vi "STD Cal Data_etc.vi"(8 "error in":errorcluster caption="에러 입력(에러 없음)", 9 "Data in":string[][](array[string]), 10 "문자열":string, 11 "Func_ext":string) -> (0 "error out":errorcluster caption="에러 출력", 1 "Data Out":string[][](array[string]), 3 "Func_ext Out":string, 4 "Data Out 2":string[](array[string]), 6 "Cal STD":string[][](array[string]))   [LabVIEW 2020]
uses:
  Controls/Cmd_Var Data IO.ctl
  Controls/Cmd_File path.ctl
  Controls/Cmd_File Type.ctl
  Variables/Global_Cal STD.vi
  Variables/Global_Cal Info.vi
  Public/Polymorph/Array Dedup_2D Str.vi
  Public/Polymorph/Data Class_2D Str.vi
  Public/Polymorph/Sort_2D Str.vi
  <vilib>/Utility/file.llb/Read Delimited Spreadsheet (string).vi
  Public/Polymorph/Array Dedup_1D Str.vi
panel:
  out "Cal STD in":string[][](array[string])
  out "Condition Default":string[][](array[string])
  out "데이터오류?":bool
  out "생성오류?":bool
  out "Condition":string[][](array[string])
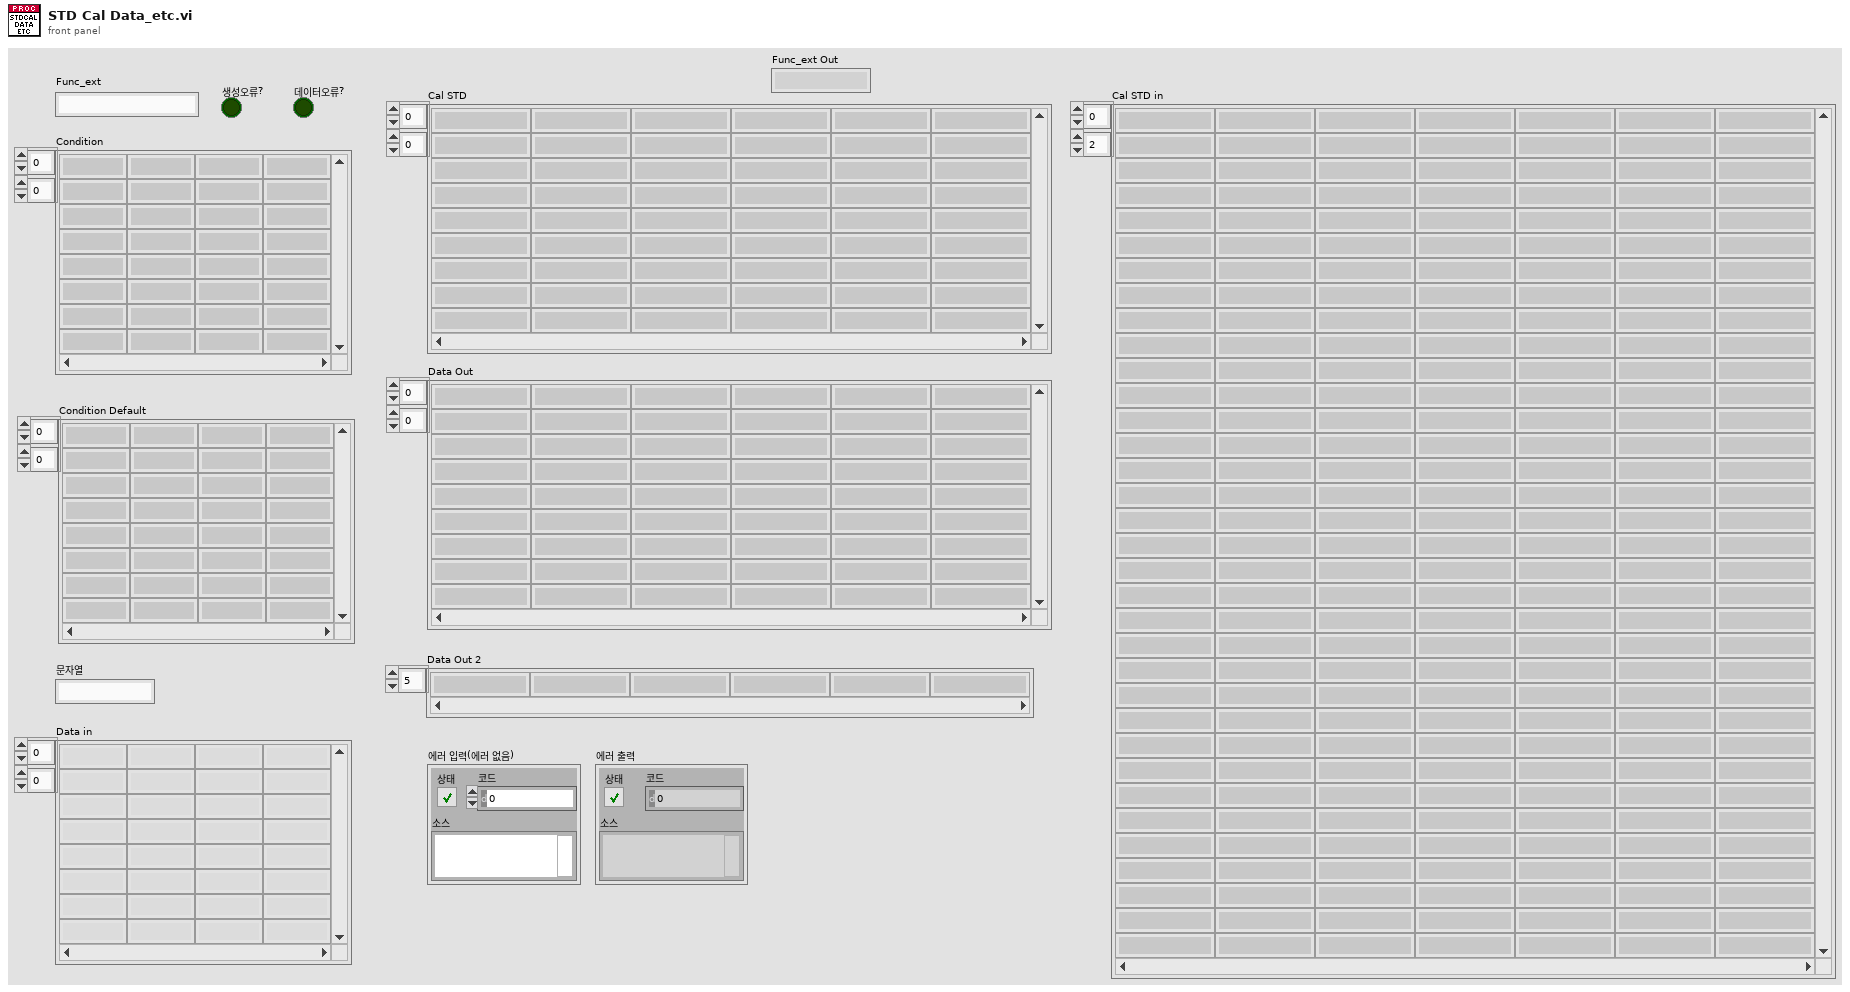
[diagram p1: front panel]
types:
  T1 = typedef "Cmd_Var Data IO.ctl" = enum16{"Condition", "Condition Default", "Condition_Temp", "Resolution", "Resolution Default", "Resolution Old", "Spec", "Spec Default", "Spec Old", "Spec Temp", "Result", "Result2", "Result3", "Result_Temp", "Result_ADJ", "Result_ADJ2", "STD1", "STD2", "STD3", "STD4", "STD5", "STD Temp", "CMC", "CMC Default"}
  T2 = cluster{"세부분류코드":string, "형식":string, "옵션":string, "측정기명":string, "EXCEL파일명":string, "TEMP":string}
  T3 = typedef "Cmd_File Type.ctl" = enum16{"엑셀", "엑셀(2003)", "텍스트", "설정", "2진", "VI", "CSV", "LOG", "폴더"}
  T4 = typedef "Cmd_File path.ctl" = enum16{"에러로그", "데이터파일경로", "성적서원본", "지난성적서", "Data Files", "경로생성", "Updater", "Template", "설정파일경로", "FTP Upload", "Update 경로", "어플리케이션"}
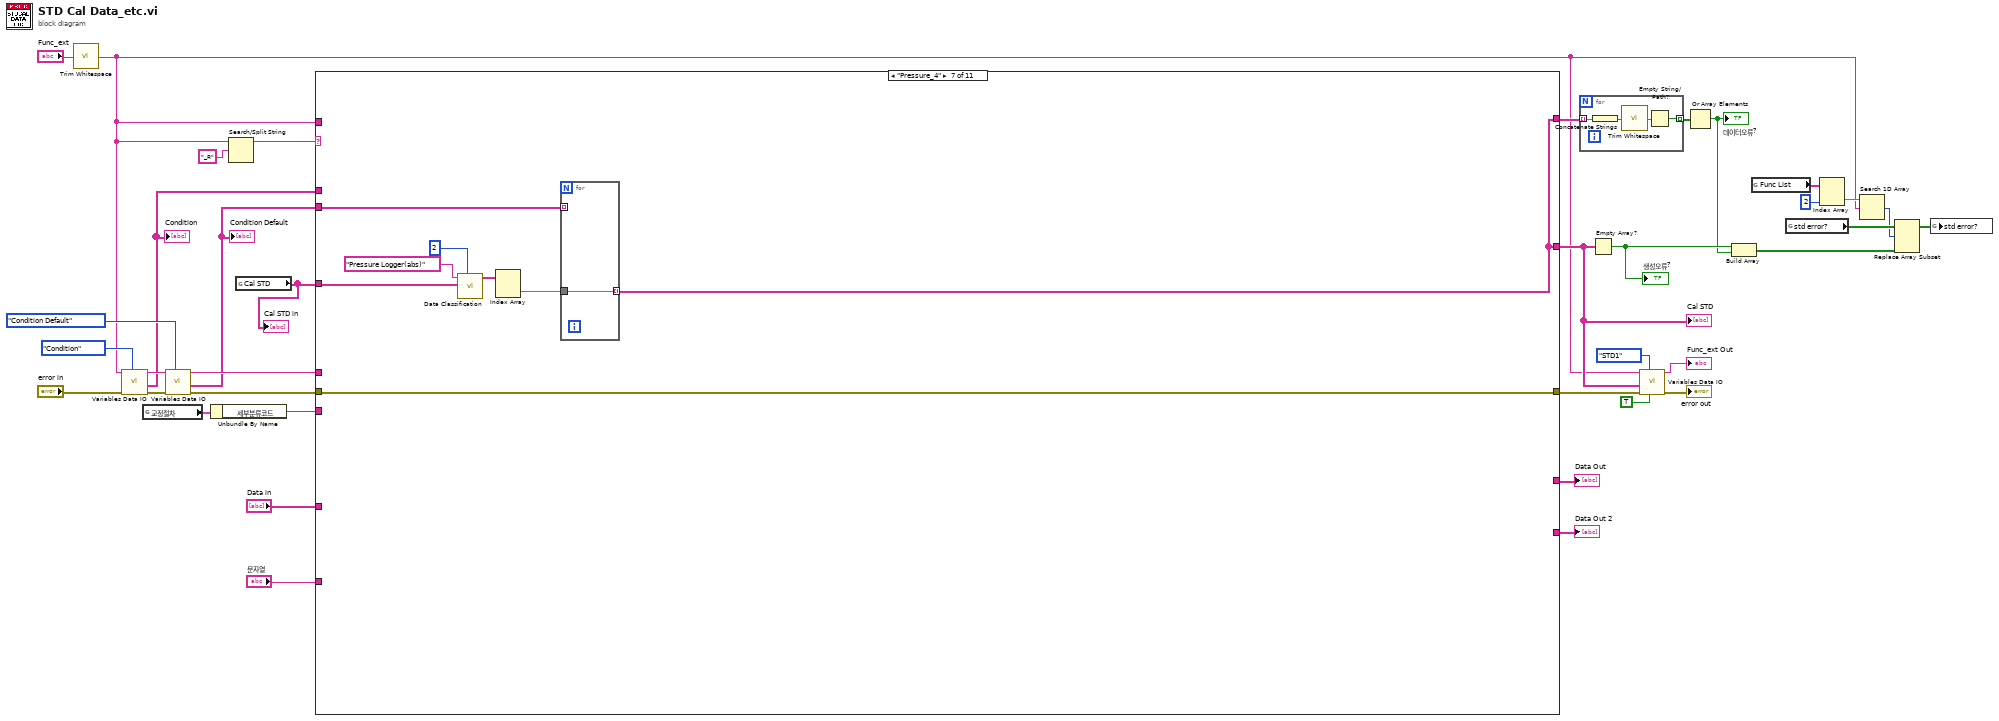
[diagram p0: block diagram]
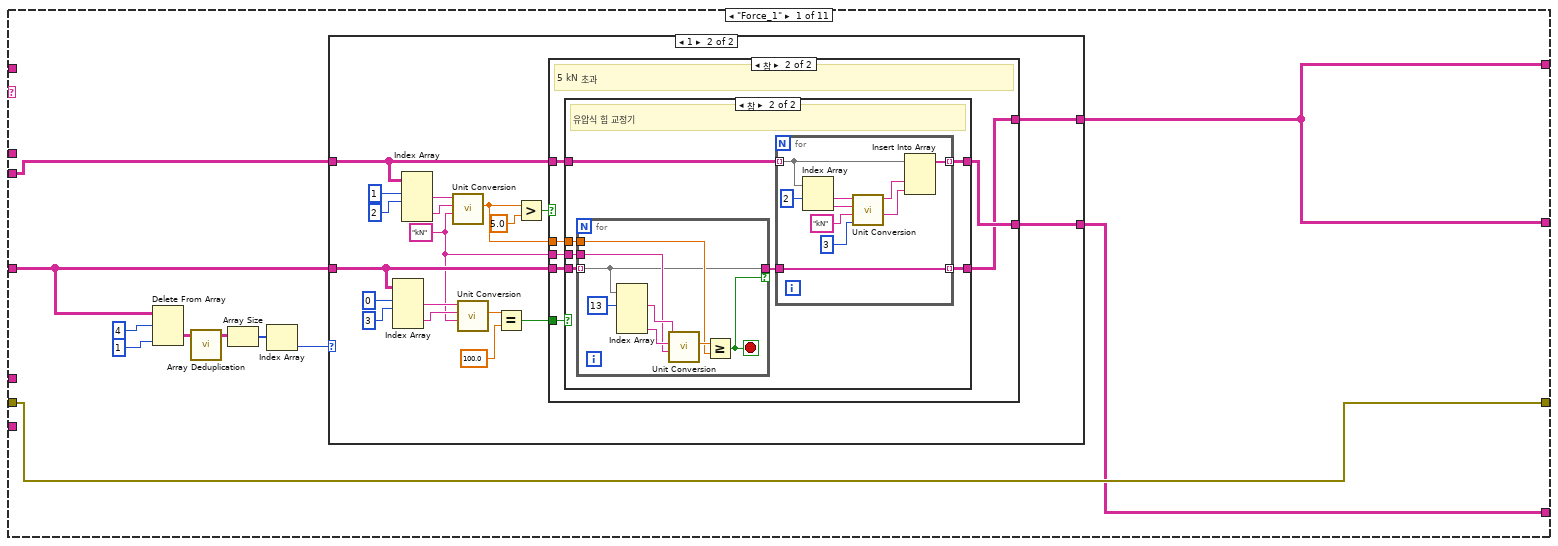
[diagram p2: hidden frame]
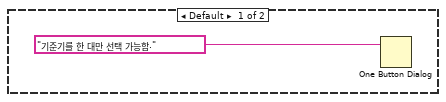
[diagram p3: hidden frame]
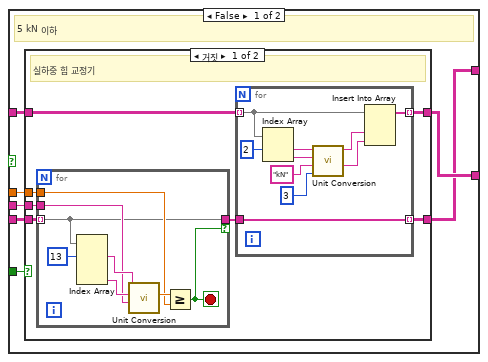
[diagram p4: hidden frame]
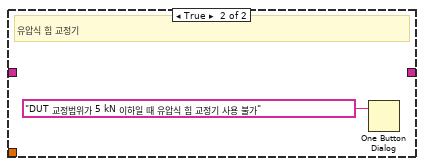
[diagram p5: hidden frame]
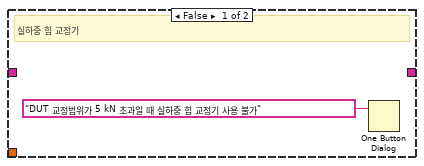
[diagram p6: hidden frame]
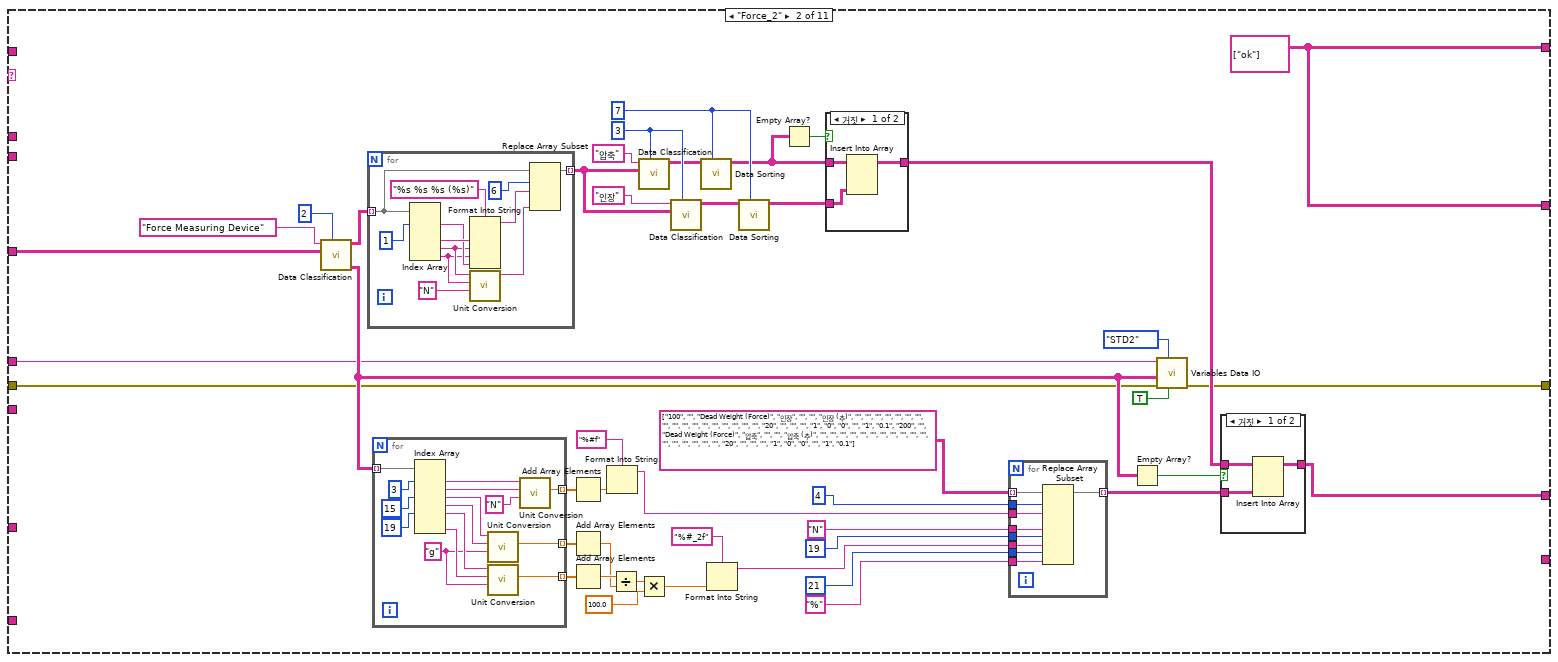
[diagram p7: hidden frame]
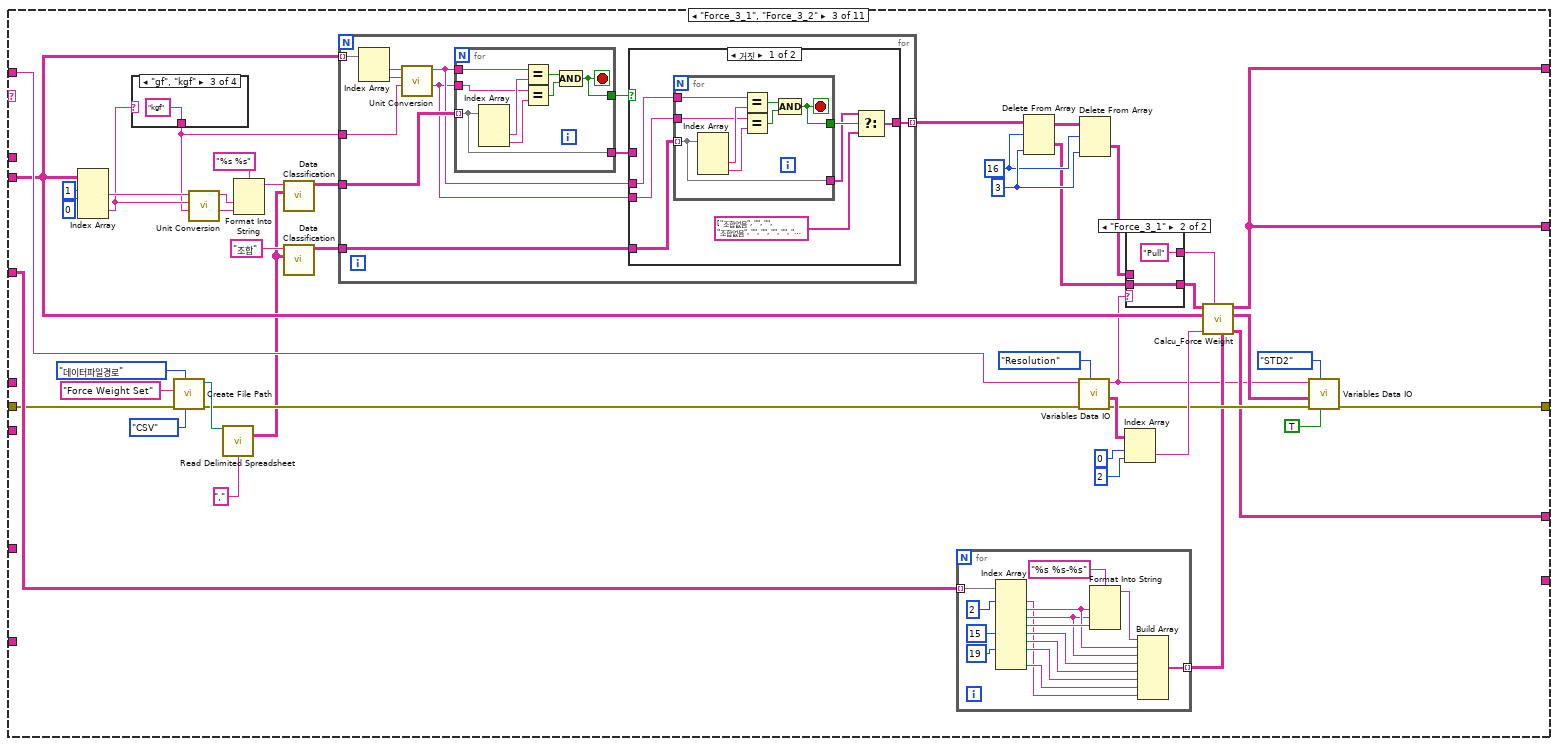
[diagram p10: hidden frame]
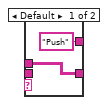
[diagram p11: hidden frame]
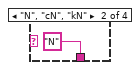
[diagram p14: hidden frame]
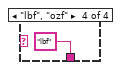
[diagram p15: hidden frame]
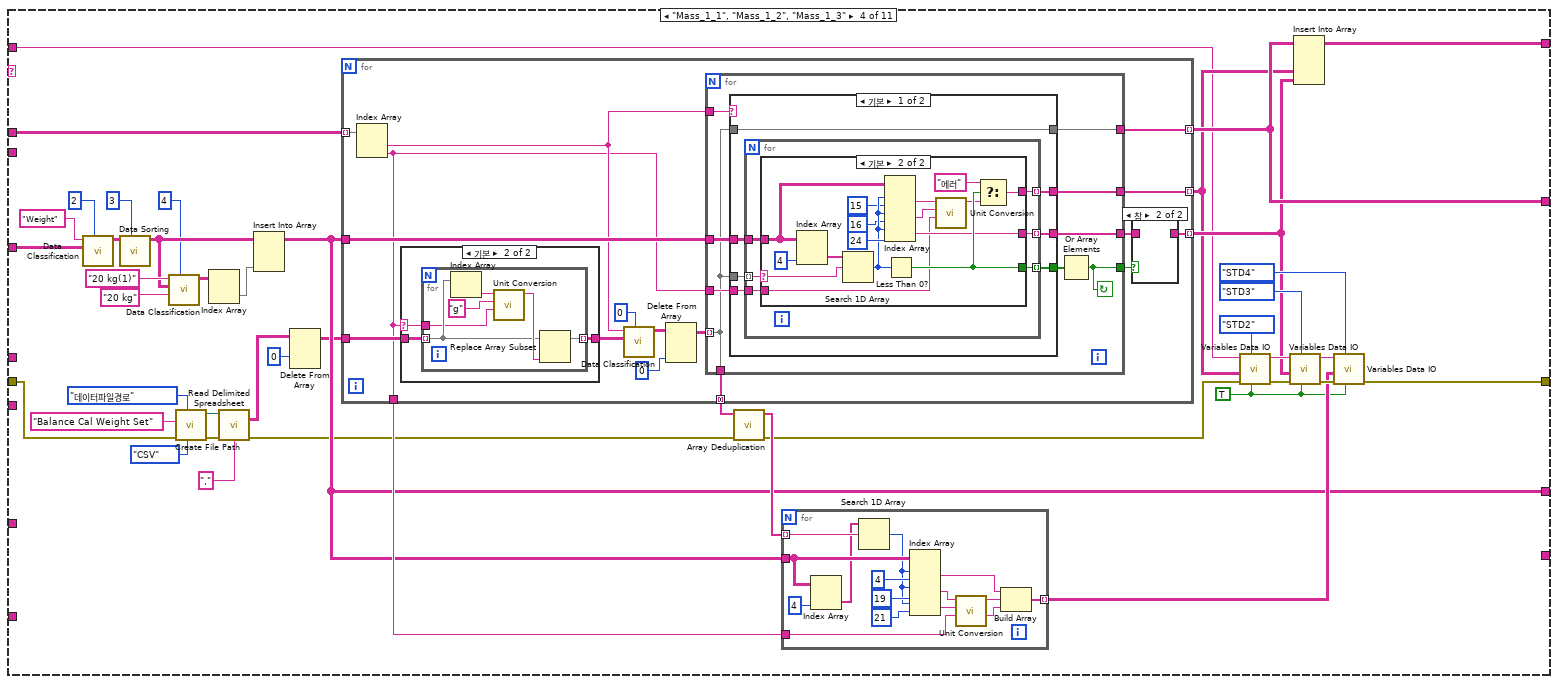
[diagram p16: hidden frame]
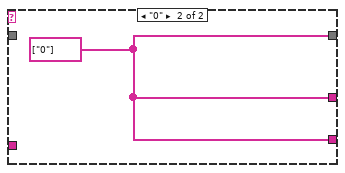
[diagram p19: hidden frame]
diagram:
  n1 = call <vilib>:"Trim Whitespace.vi"("string"="Func_ext") -> ("trimmed string"=w2:string)  [unwired: 1 in]
  n2 = call "Variables Data IO.vi"("Select"=Cmd_Var_Data_IO."Condition", "error in"="error in", "Func_ext"=w2) -> ("error out"=w24:errorcluster, "Data Out"=w9:string[][], "Func_ext Out"=w22:string)  [unwired: 6 in]
  "Condition" <- w9
  n3 = global read "Global_Cal Info.vi" "교정절차"() -> (w7:T2)
  n4 = call "Variables Data IO.vi"("Select"=Cmd_Var_Data_IO."Condition Default", "error in"=w24, "Func_ext"=w22) -> ("error out"=w23:errorcluster, "Data Out"=w8:string[][], "Func_ext Out"=w21:string)  [unwired: 6 in]
  "Condition Default" <- w8
  n5 = Unbundle By Name(w7) -> ("세부분류코드"=w6:string)
  n6 = Search/Split String(string=w2, search string/char (-)="_R" ("검색 문자열/문자 (-)")) -> (substring before match=w19:string)  [unwired: 1 in, 2 out]
  n7 = global read "Global_Cal STD.vi" "Cal STD"() -> (w37:string[][])
  "Cal STD in" <- w37
  n8 = case shown="\"Pressure_4\"" w19 {
    selector: w19 -> [_ _ _ _ _ w590 _ _ _ _ _]
    tunnel: w23 -> [w48 w149 w224 w331 w465 w598 w1082 w1101 w1192 w1315 w1342]
    tunnel: [w48 w154 w240 w351 w466 w596 w1082 w1099 w1217 w1314 w1342] -> w36
    tunnel: w37 -> [w41 w170 w258 w367 w469 w595 w1088 w1102 w1230 w1281 _]
    tunnel: [w47 w156 w233 w346 w449 w599 w1083 w1092 w1211 w1316 w1341] -> w27
    tunnel: [w45 w163 w234 w336 w462 w592 _ w1093 w1207 _ _] -> w33
    tunnel: w9 -> [_ _ _ w327 w460 _ _ w1100 _ _ _]
    tunnel: [w47 w156 w233 w344 w449 w599 w1083 w1092 w1211 w1316 w1341] -> w26
    tunnel: w8 -> [w46 _ w249 _ _ w594 w1085 _ w1233 w1279 _]
    tunnel: w21 -> [_ w152 _ _ _ w597 _ _ w1206 w1313 _]
    tunnel: w2 -> [_ _ w254 w335 w458 _ _ w1091 _ _ _]
    tunnel: w6 -> [_ _ _ _ _ w593 _ _ _ _ _]
    tunnel: [_ _ _ _ _ w591 _ _ _ w1272 string[] []] -> w5
    tunnel: "Data in" -> [_ _ _ _ _ w589 _ _ _ _ _]
    tunnel: "문자열" -> [_ _ _ _ _ _ _ _ _ _ _]
    frame "Force_1" {
      n9 = Delete From Array(array=w41, length=4 ("길이"), index (col)=1 ("비활성화된 인덱스 (열)")) -> (deleted portion=w40:string[][])  [unwired: 1 in, 1 out]
      n10 = call-poly "Array Deduplication.vi"("배열 in"=w40) -> ("배열 out"=w42:string[][])  [unwired: 9 in, 1 out]
      n11 = Array Size(array=w42) -> (size(s)=w44:i32[])
      n12 = Index Array(array=w44) -> (element=w43:i32)  [unwired: 1 in]
      n13 = case shown="1" w43 {
        tunnel: [_ w68] -> w47
        tunnel: w46 -> [_ w67]
        tunnel: w41 -> [_ w58]
        tunnel: [_ w53] -> w45
        frame Default {
          n14 = One Button Dialog(message="기준기를 한 대만 선택 가능함.") -> ()  [unwired: 1 in, 1 out]
        }
        frame 1 {
          w54 = "kN" ("환산단위")
          n15 = Index Array(array=w58, index (row) #1=0 ("비활성화된 인덱스 (행)"), index (col) #1=3 ("비활성화된 인덱스 (열)")) -> (element #1=w56:string, element #2=w57:string)  [unwired: 2 in]
          n16 = Index Array(array=w67, index (row) #1=1 ("인덱스 (행)"), index (col) #1=2 ("비활성화된 인덱스 (열)")) -> (element #1=w64:string, element #2=w63:string)  [unwired: 2 in]
          n17 = call "Unit Conversion.vi"("환산단위"=w54, "입력단위"=w63, "입력값"=w64) -> ("환산값 (DBL)"=w55:dbl)  [unwired: 3 in, 5 out]
          n18 = call "Unit Conversion.vi"("환산단위"=w54, "입력단위"=w57, "입력값"=w56) -> ("환산값 (DBL)"=w52:dbl)  [unwired: 3 in, 5 out]
          n19 = Equal?(x=w52, y=100.0) -> (x = y?=w50:bool)
          n20 = Greater?(x=w55, y=5.0) -> (0:w61:bool)
          n21 = case shown="참" w61 {
            tunnel: [w70 w103] -> w68
            tunnel: w67 -> [w75 w108]
            tunnel: w58 -> [w74 w107]
            tunnel: w55 -> [w73 w106]
            tunnel: w54 -> [w72 w105]
            tunnel: [w71 w104] -> w53
            tunnel: w50 -> [w69 w102]
            frame False {
              # "5 kN 이하"
              n22 = case shown="거짓" w69 {
                tunnel: [w82 _] -> w71
                tunnel: w75 -> [w81 _]
                tunnel: w74 -> [w80 _]
                tunnel: w73 -> [w79 _]
                tunnel: w72 -> [w78 _]
                tunnel: [w76 _] -> w70
                frame False {
                  # "실하중 힘 교정기"
                  n23 = for {
                    tunnel: w80 -> [w84] mode=indexing
                    tunnel: w79 -> [w85]
                    tunnel: w78 -> [w87]
                    tunnel: [w84] -> w77 if=w83
                    stop <- w83 stop-if-true
                    n24 = Index Array(array=w84, index #1=13 ("인덱스")) -> (element #1=w89:string, element #4=w88:string)  [unwired: 3 in, 2 out]
                    n25 = call "Unit Conversion.vi"("환산단위"=w87, "입력단위"=w88, "입력값"=w89) -> ("환산값 (DBL)"=w86:dbl)  [unwired: 3 in, 5 out]
                    n26 = Greater Or Equal?(x=w86, y=w85) -> (x >= y?=w83:bool)
                  }
                  n27 = for {
                    tunnel: w81 -> [w100] mode=indexing
                    tunnel: [w97] -> w82 mode=indexing
                    tunnel: w77 -> [w95]
                    tunnel: [w95] -> w76 mode=indexing
                    n28 = Index Array(array=w100, index #1=2 ("인덱스")) -> (element #1=w96:string, element #2=w93:string)  [unwired: 1 in]
                    n29 = call "Unit Conversion.vi"("소수점 자리수"=3, "환산단위"="kN", "입력단위"=w93, "입력값"=w96) -> ("환산단위"=w98:string, "환산값 (string)"=w99:string)  [unwired: 2 in, 4 out]
                    n30 = Insert Into Array(array=w100, new element #1=w99, new element #2=w98) -> (w97:string[])  [unwired: 1 in]
                  }
                }
                frame True {
                  # "유압식 힘 교정기"
                  n31 = One Button Dialog(message="DUT 교정범위가 5 kN 이하일 때 유압식 힘 교정기 사용 불가") -> ()  [unwired: 1 in, 1 out]
                }
              }
            }
            frame True {
              # "5 kN 초과"
              n32 = case shown="참" w102 {
                tunnel: [_ w116] -> w104
                tunnel: w108 -> [_ w115]
                tunnel: w107 -> [_ w114]
                tunnel: w106 -> [_ w113]
                tunnel: w105 -> [_ w112]
                tunnel: [_ w110] -> w103
                frame False {
                  # "실하중 힘 교정기"
                  n33 = One Button Dialog(message="DUT 교정범위가 5 kN 초과일 때 실하중 힘 교정기 사용 불가") -> ()  [unwired: 1 in, 1 out]
                }
                frame True {
                  # "유압식 힘 교정기"
                  n34 = for {
                    tunnel: w114 -> [w118] mode=indexing
                    tunnel: w113 -> [w119]
                    tunnel: w112 -> [w121]
                    tunnel: [w118] -> w111 if=w117
                    stop <- w117 stop-if-true
                    n35 = Index Array(array=w118, index #1=13 ("인덱스")) -> (element #1=w123:string, element #4=w122:string)  [unwired: 3 in, 2 out]
                    n36 = call "Unit Conversion.vi"("환산단위"=w121, "입력단위"=w122, "입력값"=w123) -> ("환산값 (DBL)"=w120:dbl)  [unwired: 3 in, 5 out]
                    n37 = Greater Or Equal?(x=w120, y=w119) -> (x >= y?=w117:bool)
                  }
                  n38 = for {
                    tunnel: w115 -> [w134] mode=indexing
                    tunnel: [w131] -> w116 mode=indexing
                    tunnel: w111 -> [w129]
                    tunnel: [w129] -> w110 mode=indexing
                    n39 = Index Array(array=w134, index #1=2 ("인덱스")) -> (element #1=w130:string, element #2=w127:string)  [unwired: 1 in]
                    n40 = call "Unit Conversion.vi"("소수점 자리수"=3, "환산단위"="kN", "입력단위"=w127, "입력값"=w130) -> ("환산단위"=w132:string, "환산값 (string)"=w133:string)  [unwired: 2 in, 4 out]
                    n41 = Insert Into Array(array=w134, new element #1=w133, new element #2=w132) -> (w131:string[])  [unwired: 1 in]
                  }
                }
              }
            }
          }
        }
      }
    }
    frame "Force_2" {
      w177 = 3 ("인덱스")
      w178 = u16 7 ("기준열")
      w156 = string[][] [["ok"]] ("Data out")
      n42 = call-poly "Data Classification.vi"("인덱스"=2, "DATA 입력"=w170, "검색 문자열"="Force Measuring Device") -> ("제외 DATA 출력"=w153:string[][], "DATA 출력"=w169:string[][])  [unwired: 4 in, 3 out]
      n43 = for {
        tunnel: w169 -> [w220] mode=indexing
        tunnel: [w217] -> w171 mode=indexing
        n44 = Index Array(array=w220, index #1=1 ("인덱스")) -> (element #1=w215:string, element #3=w222:string, element #4=w214:string, element #5=w213:string)  [unwired: 4 in, 1 out]
        n45 = Format Into String(format string="%s %s %s (%s)" ("포맷 문자열"), w222, w214, w213, w215) -> (resulting string=w218:string)  [unwired: 2 in, 1 out]
        n46 = call "Unit Conversion.vi"("환산단위"="N", "입력단위"=w213, "입력값"=w214) -> ("환산값 (string)"=w211:string)  [unwired: 3 in, 5 out]
        n47 = Replace Array Subset(array=w220, new element #1=w218, index #1=6 ("인덱스"), new element #2=w211) -> (w217:string[])  [unwired: 1 in]
      }
      n48 = for {
        tunnel: w153 -> [w201] mode=indexing
        tunnel: [w197] -> w162 mode=indexing
        tunnel: [w189] -> w148 mode=indexing
        tunnel: [w188] -> w147 mode=indexing
        w190 = "g" ("환산단위")
        n49 = Index Array(array=w201, index #1=3 ("인덱스"), index #3=15 ("인덱스"), index #5=19 ("인덱스")) -> (element #1=w199:string, element #2=w198:string, element #3=w195:string, element #4=w194:string, element #5=w192:string, element #7=w191:string)  [unwired: 4 in, 1 out]
        n50 = call "Unit Conversion.vi"("환산단위"=w190, "입력단위"=w194, "입력값"=w195) -> ("환산값 (DBL)"=w189:dbl)  [unwired: 3 in, 5 out]
        n51 = call "Unit Conversion.vi"("환산단위"=w190, "입력단위"=w191, "입력값"=w192) -> ("환산값 (DBL)"=w188:dbl)  [unwired: 3 in, 5 out]
        n52 = call "Unit Conversion.vi"("환산단위"="N", "입력단위"=w198, "입력값"=w199) -> ("환산값 (DBL)"=w197:dbl)  [unwired: 3 in, 5 out]
      }
      n53 = Add Array Elements(numeric array=w162) -> (sum=w161:dbl)
      n54 = Add Array Elements(numeric array=w148) -> (sum=w145:dbl)
      n55 = Add Array Elements(numeric array=w147) -> (sum=w146:dbl)
      n56 = Format Into String(format string="%#f" ("포맷 문자열"), w161) -> (resulting string=w159:string)  [unwired: 2 in, 1 out]
      n57 = Divide(x=w146, y=w145) -> (x/y=w144:dbl)
      n58 = call-poly "Data Classification.vi"("인덱스"=w177, "DATA 입력"=w171, "검색 문자열"="압축") -> ("DATA 출력"=w172:string[][])  [unwired: 4 in, 4 out]
      n59 = Multiply(x=w144, y=100.0) -> (x*y=w141:dbl)
      n60 = call-poly "Data Classification.vi"("인덱스"=w177, "DATA 입력"=w171, "검색 문자열"="인장") -> ("DATA 출력"=w175:string[][])  [unwired: 4 in, 4 out]
      n61 = call-poly "Data Sorting.vi"("기준열"=w178, "Data in"=w172) -> ("Data out"=w166:string[][])  [unwired: 8 in, 1 out]
      n62 = Format Into String(format string="%#_2f" ("포맷 문자열"), w141) -> (resulting string=w140:string)  [unwired: 2 in, 1 out]
      n63 = call-poly "Data Sorting.vi"("기준열"=w178, "Data in"=w175) -> ("Data out"=w176:string[][])  [unwired: 8 in, 1 out]
      n64 = Empty Array?(array=w166) -> (empty?=w165:bool)
      n65 = case shown="거짓" w165 {
        tunnel: w176 -> [w209 w210]
        tunnel: [w208 w210] -> w164
        tunnel: w166 -> [w207 _]
        frame False {
          n66 = Insert Into Array(array=w207, new element=w209) -> (w208:string[][])  [unwired: 2 in]
        }
        frame True {
        }
      }
      n67 = for {
        tunnel: string[][] [["100", "", "Dead Weight (Force)", "인장", "", "", "인장 (추)", "", "", "", "", "", "", "", "", "", "", "", "", "", "", "", "", "", "20", "", "", "", "1", "0", "0", "", "1", "0.1"], ["200", "", "Dead Weight (Force)", "압축", "", "", "압축 (추)", "", "", "", "", "", "", "", "", "", "", "", "", "", "", "", "", "", "20", "", "", "", "1", "0", "0", "", "1", "0.1"]] -> [w187] mode=indexing
        tunnel: w159 -> [w186]
        tunnel: [w185] -> w158 mode=indexing
        tunnel: "N" ("새 원소/부분배열") -> [w184]
        tunnel: 19 ("인덱스") -> [w183]
        tunnel: w140 -> [w182]
        tunnel: 21 ("인덱스") -> [w181]
        tunnel: "%" ("새 원소/부분배열") -> [w180]
        tunnel: 4 ("인덱스") -> [w179]
        n68 = Replace Array Subset(array=w187, new element #1=w186, index #1=w179, new element #2=w184, new element #3=w182, index #3=w183, new element #4=w180, index #4=w181) -> (w185:string[])  [unwired: 1 in]
      }
      n69 = Empty Array?(array=w153) -> (empty?=w151:bool)
      n70 = call "Variables Data IO.vi"("Write blank data ?(F)"=TRUE ("Write blank data ?(T)"), "Select"=Cmd_Var_Data_IO."STD2", "error in"=w149, "Data In"=w153, "Func_ext"=w152) -> ("error out"=w154:errorcluster)  [unwired: 4 in, 2 out]
      n71 = case shown="거짓" w151 {
        tunnel: [w205 w206] -> w163
        tunnel: w164 -> [w204 w206]
        tunnel: w158 -> [w203 _]
        frame False {
          n72 = Insert Into Array(array=w204, new element=w203) -> (w205:string[][])  [unwired: 2 in]
        }
        frame True {
        }
      }
    }
    frame "Force_3_1", "Force_3_2" {
      w245 = 16 ("길이")
      w246 = 3 ("비활성화된 인덱스 (열)")
      n73 = Index Array(array=w249, index (row) #1=1 ("인덱스 (행)"), index (col) #1=0 ("비활성화된 인덱스 (열)")) -> (element #1=w265:string, element #2=w264:string)  [unwired: 2 in]
      n74 = case shown="\"gf\", \"kgf\"" w264 {
        tunnel: [_ "N" "kgf" "lbf"] -> w257
        frame Default {
        }
        frame "N", "cN", "kN" {
        }
        frame "gf", "kgf" {
        }
        frame "lbf", "ozf" {
        }
      }
      n75 = call "Create File Path.vi"("파일타입"=Cmd_File_Type."CSV", "항목"=Cmd_File_path."데이터파일경로", "에러 입력"=w224, "문자열 in"="Force Weight Set" ("delimiter (\\t)")) -> ("error out"=w225:errorcluster, "파일경로"=w226:path)  [unwired: 4 in, 2 out]
      n76 = call "Unit Conversion.vi"("환산단위"=w257, "입력단위"=w264, "입력값"=w265) -> ("환산단위"=w262:string, "환산값 (string)"=w263:string)  [unwired: 3 in, 4 out]
      n77 = call-poly <vilib>:"Read Delimited Spreadsheet.vi"("file path (dialog if empty)"=w226, "delimiter (\\t)"="," ("delimiter (\\t)")) -> ("all rows"=w223:string[][])  [unwired: 8 in, 5 out]
      n78 = Format Into String(format string="%s %s" ("포맷 문자열"), w263, w262) -> (resulting string=w260:string)  [unwired: 2 in, 1 out]
      n79 = call-poly "Data Classification.vi"("DATA 입력"=w223, "검색 문자열"=w260) -> ("DATA 출력"=w230:string[][])  [unwired: 5 in, 4 out]
      n80 = call-poly "Data Classification.vi"("DATA 입력"=w223, "검색 문자열"="조합") -> ("DATA 출력"=w231:string[][])  [unwired: 5 in, 4 out]
      n81 = for {
        tunnel: w249 -> [w282] mode=indexing
        tunnel: w257 -> [w278]
        tunnel: w230 -> [w281]
        tunnel: w231 -> [w274]
        tunnel: [w275] -> w255 mode=indexing
        n82 = Index Array(array=w282) -> (element #1=w280:string, element #2=w279:string)  [unwired: 2 in]
        n83 = call "Unit Conversion.vi"("환산단위"=w278, "입력단위"=w279, "입력값"=w280) -> ("환산단위"=w272:string, "환산값 (string)"=w273:string)  [unwired: 3 in, 4 out]
        n84 = for {
          tunnel: w281 -> [w300] mode=indexing
          tunnel: w273 -> [w306]
          tunnel: w272 -> [w304]
          tunnel: [w300] -> w276
          tunnel: [w299] -> w277
          stop <- w299 stop-if-true
          n85 = Index Array(array=w300) -> (element #2=w305:string, element #3=w303:string)  [unwired: 3 in, 1 out]
          n86 = Equal?(x=w306, y=w305) -> (x = y?=w302:bool)
          n87 = Equal?(x=w304, y=w303) -> (x = y?=w301:bool)
          n88 = Compound Arithmetic op=AND(w302, w301) -> (w299:bool)
        }
        n89 = case shown="거짓" w277 {
          tunnel: w276 -> [_ w298]
          tunnel: [w284 w298] -> w275
          tunnel: w274 -> [w289 _]
          tunnel: w273 -> [w288 _]
          tunnel: w272 -> [w287 _]
          frame False {
            n90 = for {
              tunnel: w289 -> [w291] mode=indexing
              tunnel: w288 -> [w297]
              tunnel: w287 -> [w295]
              tunnel: [w291] -> w285
              tunnel: [w290] -> w286
              stop <- w290 stop-if-true
              n91 = Index Array(array=w291) -> (element #2=w296:string, element #3=w294:string)  [unwired: 3 in, 1 out]
              n92 = Equal?(x=w297, y=w296) -> (x = y?=w293:bool)
              n93 = Equal?(x=w295, y=w294) -> (x = y?=w292:bool)
              n94 = Compound Arithmetic op=AND(w293, w292) -> (w290:bool)
            }
            n95 = Select(t=w285, s=w286, f=string[] ["조합없음", "", "", "조합없음", "", "", "", "", "", "", "", "", "", "", "", "", "", "", "", "조합없음"]) -> (s? t:f=w284:string[])
          }
          frame True {
          }
        }
      }
      n96 = for {
        tunnel: w258 -> [w318] mode=indexing
        tunnel: [w317] -> w235 mode=indexing
        n97 = Index Array(array=w318, index #1=2 ("인덱스"), index #5=15 ("인덱스"), index #7=19 ("인덱스")) -> (element #1=w307:string, element #2=w310:string, element #3=w309:string, element #4=w321:string, element #5=w315:string, element #6=w314:string, element #7=w312:string, element #9=w311:string)  [unwired: 6 in, 1 out]
        n98 = Format Into String(format string="%s %s-%s" ("포맷 문자열"), w310, w309, w321) -> (resulting string=w319:string)  [unwired: 2 in, 1 out]
        n99 = Build Array(w319, w310, w309, w315, w314, w312, w311, w307) -> (w317:string[])
      }
      n100 = Delete From Array(array=w255, length=w245, index (col)=w246) -> (deleted portion=w238:string[][], array with subset deleted=w247:string[][])  [unwired: 1 in]
      n101 = call "Variables Data IO.vi"("Select"=Cmd_Var_Data_IO."Resolution", "error in"=w225, "Func_ext"=w254) -> ("error out"=w243:errorcluster, "Data Out"=w252:string[][], "Func_ext Out"=w232:string)  [unwired: 6 in]
      n102 = Delete From Array(array=w247, length=w245, index (col)=w246) -> (deleted portion=w236:string[][])  [unwired: 1 in, 1 out]
      n103 = Index Array(array=w252, index (row)=0 ("인덱스 (행)"), index (col)=2 ("비활성화된 인덱스 (열)")) -> (element=w248:string)
      n104 = case shown="\"Force_3_1\"" w232 {
        tunnel: ["Push" ("방향") "Pull" ("방향")] -> w239
        tunnel: w238 -> [_ w270]
        tunnel: [w268 w270] -> w237
        tunnel: w236 -> [w268 _]
        frame Default {
        }
        frame "Force_3_1" {
        }
      }
      n105 = call "Calcu_Force Weight.vi"("기준기 데이터"=w235, "방향"=w239, "분해능"=w248, "Condition"=w249, "분동조합"=w237) -> ("Condition Out"=w234:string[][], "사용기준추"=w242:string[][], "기준추 데이터"=w233:string[][])  [unwired: 3 in, 1 out]
      n106 = call "Variables Data IO.vi"("Write blank data ?(F)"=TRUE ("Write blank data ?(T)"), "Select"=Cmd_Var_Data_IO."STD2", "error in"=w243, "Data In"=w242, "Func_ext"=w232) -> ("error out"=w240:errorcluster)  [unwired: 4 in, 2 out]
    }
    frame "Mass_1_1", "Mass_1_2", "Mass_1_3" {
      w348 = TRUE ("Write blank data ?(T)")
      n107 = call-poly "Data Classification.vi"("인덱스"=2, "DATA 입력"=w367, "검색 문자열"="Weight") -> ("DATA 출력"=w364:string[][])  [unwired: 4 in, 4 out]
      n108 = call-poly "Data Sorting.vi"("기준열"=u16 3, "Data in"=w364) -> ("Data out"=w341:string[][])  [unwired: 8 in, 1 out]
      n109 = call-poly "Data Classification.vi"("인덱스"=4, "대체 문자열"="20 kg" ("검색 문자열"), "DATA 입력"=w341, "검색 문자열"="20 kg(1)") -> ("DATA 출력"=w342:string[][])  [unwired: 3 in, 4 out]
      n110 = call "Create File Path.vi"("파일타입"=Cmd_File_Type."CSV", "항목"=Cmd_File_path."데이터파일경로", "에러 입력"=w331, "문자열 in"="Balance Cal Weight Set" ("delimiter (\\t)")) -> ("error out"=w326:errorcluster, "파일경로"=w330:path)  [unwired: 4 in, 2 out]
      n111 = Index Array(array=w342) -> (element=w340:string[])  [unwired: 2 in]
      n112 = call-poly <vilib>:"Read Delimited Spreadsheet.vi"("file path (dialog if empty)"=w330, "error in (no error)"=w326, "delimiter (\\t)"="," ("delimiter (\\t)")) -> ("all rows"=w329:string[][], "error out"=w325:errorcluster)  [unwired: 7 in, 4 out]
      n113 = Insert Into Array(array=w341, new element=w340) -> (w336:string[][])  [unwired: 2 in]
      n114 = Delete From Array(array=w329, index (row)=0 ("인덱스 (행)")) -> (array with subset deleted=w328:string[][])  [unwired: 2 in, 1 out]
      n115 = for {
        tunnel: [w394] -> w346 mode=indexing
        tunnel: [w389] -> w359 mode=concatenating
        tunnel: w336 -> [w398]
        tunnel: [w393] -> w337 mode=indexing
        tunnel: [w395] -> w345 mode=indexing
        tunnel: [w383] -> w347
        tunnel: w328 -> [w385]
        tunnel: w327 -> [w387] mode=indexing
        n116 = Index Array(array=w387) -> (element #1=w386:string, element #2=w383:string)  [unwired: 2 in]
        n117 = case shown="기본" w383 {
          selector: w383 -> [_ w400]
          tunnel: w385 -> [w399 w402]
          tunnel: [w399 w401] -> w384
          frame "g" {
          }
          frame Default {
            n118 = for {
              tunnel: w402 -> [w404] mode=indexing
              tunnel: [w408] -> w401 mode=indexing
              tunnel: w400 -> [w403]
              n119 = Index Array(array=w404) -> (element=w407:string)  [unwired: 1 in]
              n120 = call "Unit Conversion.vi"("환산단위"=w403, "입력단위"="g", "입력값"=w407) -> ("환산값 (string)"=w405:string)  [unwired: 3 in, 5 out]
              n121 = Replace Array Subset(array=w404, new element=w405) -> (w408:string[])  [unwired: 1 in]
            }
          }
        }
        n122 = call-poly "Data Classification.vi"("인덱스"=0, "DATA 입력"=w384, "검색 문자열"=w386) -> ("DATA 출력"=w392:string[][])  [unwired: 4 in, 4 out]
        n123 = Delete From Array(array=w392, index (col)=0 ("인덱스")) -> (array with subset deleted=w390:string[][])  [unwired: 2 in, 1 out]
        n124 = for {
          tunnel: w398 -> [w417]
          tunnel: [w410] -> w397
          tunnel: [w415] -> w396
          tunnel: [w414] -> w394
          tunnel: [w413] -> w393
          tunnel: w383 -> [w412]
          tunnel: w386 -> [w411]
          tunnel: w390 -> [w409] mode=indexing
          tunnel: [w409] -> w389
          stop <- w410 continue-if-true
          n125 = case shown="기본" w411 {
            tunnel: w417 -> [w424 _]
            tunnel: [w423 w447] -> w413
            tunnel: [w422 w447] -> w415
            tunnel: w409 -> [w421 _]
            tunnel: w409 -> [w420 _]
            tunnel: [w420 w447] -> w414
            tunnel: [w419 _] -> w416
            tunnel: w412 -> [w418 _]
            frame Default {
              n126 = for {
                tunnel: w421 -> [w426] mode=indexing
                tunnel: w424 -> [w430]
                tunnel: [w429] -> w423 mode=indexing
                tunnel: [w428] -> w422 mode=indexing
                tunnel: [w427] -> w419 mode=indexing
                tunnel: w418 -> [w425]
                n127 = case shown="기본" w426 {
                  selector: w426 -> [_ w442]
                  tunnel: w430 -> [_ w444]
                  tunnel: [_ w440] -> w429
                  tunnel: [_ w433] -> w428
                  tunnel: [_ w441] -> w427
                  tunnel: w425 -> [_ w432]
                  frame "" {
                  }
                  frame Default {
                    n128 = Index Array(array=w444, index (col)=4 ("비활성화된 인덱스 (열)")) -> (element=w445:string[])  [unwired: 1 in]
                    n129 = Search 1D Array(1D array=w445, element=w442) -> (index of element=w438:i32)  [unwired: 1 in]
                    n130 = Index Array(array=w444, index (row) #1=w438, index (col) #1=15 ("비활성화된 인덱스 (열)"), index (row) #2=w438, index (col) #2=16 ("비활성화된 인덱스 (열)"), index (row) #3=w438, index (col) #3=24 ("비활성화된 인덱스 (열)")) -> (element #1=w436:string, element #2=w431:string, element #3=w433:string)
                    n131 = Less Than 0?(x=w438) -> (x < 0?=w441:bool)
                    n132 = call "Unit Conversion.vi"("환산단위"=w432, "입력단위"=w431, "입력값"=w436) -> ("환산값 (string)"=w435:string)  [unwired: 3 in, 5 out]
                    n133 = Select(t="에러", s=w441, f=w435) -> (s? t:f=w440:string)
                  }
                }
              }
            }
            frame "0" {
              w447 = string[] ["0"] ("t")
            }
          }
          n134 = Or Array Elements(Boolean array=w416) -> (logical OR=w410:bool)
        }
        n135 = case shown="참" w397 {
          tunnel: w396 -> [w448 _]
          tunnel: [w448 _] -> w395
          frame False {
          }
          frame True {
          }
        }
      }
      n136 = call-poly "Array Deduplication.vi"("error in (no error)"=w325, "배열 in"=w359) -> ("error out"=w355:errorcluster, "배열 out"=w358:string[])  [unwired: 8 in]
      n137 = for {
        tunnel: w358 -> [w382] mode=indexing
        tunnel: w336 -> [w381]
        tunnel: [w373] -> w349 mode=indexing
        tunnel: w347 -> [w370]
        n138 = Index Array(array=w381, index (col)=4 ("비활성화된 인덱스 (열)")) -> (element=w379:string[])  [unwired: 1 in]
        n139 = Search 1D Array(1D array=w379, element=w382) -> (index of element=w376:i32)  [unwired: 1 in]
        n140 = Index Array(array=w381, index (row) #1=w376, index (col) #1=4 ("비활성화된 인덱스 (열)"), index (row) #2=w376, index (col) #2=19 ("인덱스 (열)"), index (row) #3=w376, index (col) #3=21 ("비활성화된 인덱스 (열)")) -> (element #1=w374:string, element #2=w372:string, element #3=w371:string)
        n141 = call "Unit Conversion.vi"("환산단위"=w370, "입력단위"=w371, "입력값"=w372) -> ("환산단위"=w368:string, "환산값 (string)"=w369:string)  [unwired: 3 in, 4 out]
        n142 = Build Array(w374, w369, w368) -> (w373:string[])
      }
      n143 = call "Variables Data IO.vi"("Write blank data ?(F)"=w348, "Select"=Cmd_Var_Data_IO."STD2", "error in"=w355, "Data In"=w337, "Func_ext"=w335) -> ("error out"=w354:errorcluster, "Func_ext Out"=w356:string)  [unwired: 4 in, 1 out]
      n144 = call "Variables Data IO.vi"("Write blank data ?(F)"=w348, "Select"=Cmd_Var_Data_IO."STD3", "error in"=w354, "Data In"=w345, "Func_ext"=w356) -> ("error out"=w352:errorcluster, "Func_ext Out"=w350:string)  [unwired: 4 in, 1 out]
      n145 = Insert Into Array(array=w346, new element #1=w337, new element #2=w345) -> (w344:string[][])  [unwired: 2 in]
      n146 = call "Variables Data IO.vi"("Write blank data ?(F)"=w348, "Select"=Cmd_Var_Data_IO."STD4", "error in"=w352, "Data In"=w349, "Func_ext"=w350) -> ("error out"=w351:errorcluster)  [unwired: 4 in, 2 out]
    }
    frame "Mass_2_1", "Mass_2_2" {
      w459 = TRUE ("Write blank data ?(T)")
      n147 = call-poly "Data Classification.vi"("인덱스"=2, "DATA 입력"=w469, "검색 문자열"="Weight") -> ("DATA 출력"=w450:string[][])  [unwired: 4 in, 4 out]
      n148 = call-poly "Data Classification.vi"("인덱스"=2, "DATA 입력"=w469, "검색 문자열"="Electric Balance") -> ("DATA 출력"=w455:string[][])  [unwired: 4 in, 4 out]
      n149 = call-poly "Data Sorting.vi"("기준열"=u16 13, "Data in"=w455) -> ("Data out"=w451:string[][])  [unwired: 8 in, 1 out]
      n150 = for {
        tunnel: w460 -> [w535] mode=indexing
        tunnel: w450 -> [w476]
        tunnel: [w471] -> w449 mode=indexing
        tunnel: w451 -> [w530]
        tunnel: [w529] -> w467 mode=indexing
        tunnel: [w523] -> w462 mode=indexing
        tunnel: w458 -> [w499]
        w519 = "mg" ("환산단위")
        w520 = "g" ("환산단위")
        w506 = 24 ("비활성화된 인덱스 (열)")
        w501 = 21 ("비활성화된 인덱스 (열)")
        w504 = 19 ("비활성화된 인덱스 (열)")
        w509 = 15 ("비활성화된 인덱스 (열)")
        n151 = case shown="기본" w499 {
          tunnel: w535 -> [w557 w563]
          tunnel: [w548 w562] -> w531
          tunnel: [w551 w560] -> w498
          tunnel: [w549 w560] -> w497
          tunnel: [w549 w560] -> w485
          tunnel: [w548 w562] -> w483
          tunnel: ["추" ("문자열") w558] -> w477
          frame "Mass_2_2" {
            n152 = Index Array(array=w557, index #1=3 ("인덱스")) -> (element #1=w550:string, element #2=w549:string, element #3=w548:string)  [unwired: 2 in]
            n153 = Fract/Exp String To Number(string=w550) -> (number=w554:dbl)  [unwired: 3 in, 1 out]
            n154 = Fract/Exp String To Number(string=w549) -> (number=w555:dbl)  [unwired: 3 in, 1 out]
            n155 = Max & Min(x=w554, y=w555) -> (max(x,y)=w553:dbl)  [unwired: 1 out]
            n156 = Format Into String(format string="%#f" ("포맷 문자열"), w553) -> (resulting string=w551:string)  [unwired: 2 in, 1 out]
          }
          frame Default {
            n157 = Index Array(array=w563, index #1=4 ("인덱스"), index #3=1 ("인덱스")) -> (element #1=w560:string, element #2=w562:string, element #3=w558:string)  [unwired: 1 in]
          }
        }
        n158 = case shown="기본" w477 {
          tunnel: w476 -> [w539 w540 w542]
          tunnel: [w537 w540 w541] -> w475
          frame "F1" {
            n159 = call-poly "Data Classification.vi"("인덱스"=5, "DATA 입력"=w539, "검색 문자열"="E2") -> ("DATA 출력"=w537:string[][])  [unwired: 4 in, 4 out]
          }
          frame "추" {
          }
          frame Default {
            n160 = call-poly "Data Classification.vi"("인덱스"=5, "DATA 입력"=w542, "검색 문자열"="F1") -> ("DATA 출력"=w543:string[][])  [unwired: 4 in, 4 out]
            n161 = Empty Array?(array=w543) -> (empty?=w544:bool)
            n162 = Select(t=w542, s=w544, f=w543) -> (s? t:f=w541:string[][])
          }
        }
        n163 = Fract/Exp String To Number(string=w497) -> (number=w487:dbl)  [unwired: 3 in, 1 out]
        n164 = Equal?(x=w487, y=0.5) -> (x = y?=w489:bool)
        n165 = Equal?(x=w487, y=0.05) -> (x = y?=w495:bool)
        n166 = Select(t="1 g" ("원소"), s=w489, f="500 mg" ("원소")) -> (s? t:f=w486:string)
        n167 = Select(t="100 mg" ("원소"), s=w495, f="50 mg" ("원소")) -> (s? t:f=w492:string)
        n168 = for {
          tunnel: w498 -> [w588]
          tunnel: w531 -> [w568]
          tunnel: w530 -> [w581] mode=indexing
          tunnel: 16 ("비활성화된 인덱스 (열)") -> [w584]
          tunnel: 13 ("인덱스 (열)") -> [w583]
          tunnel: [w573] -> w529
          tunnel: 24 ("인덱스 (열)") -> [w580]
          tunnel: [w576] -> w527
          tunnel: 1 ("인덱스 (열)") -> [w575]
          tunnel: 34 ("인덱스 (열)") -> [w572]
          tunnel: [w570] -> w523
          tunnel: w492 -> [w565]
          tunnel: w486 -> [w564]
          stop <- w585 stop-if-true
          n169 = Index Array(array=w581, index #1=w584, index #2=w583, index #3=w580, index #4=w575, index #5=w572) -> (element #1=w569:string, element #2=w582:string, element #3=w567:string, element #4=w574:string, element #5=w571:string)
          n170 = Fract/Exp String To Number(string=w567) -> (number=w579:dbl)  [unwired: 3 in, 1 out]
          n171 = call "Unit Conversion.vi"("환산단위"=w569, "입력단위"=w568, "입력값"=w588) -> ("환산값 (DBL)"=w586:dbl)  [unwired: 3 in, 5 out]
          n172 = Fract/Exp String To Number(string=w582) -> (number=w587:dbl)  [unwired: 3 in, 1 out]
          n173 = Build Array(w574, w567, w571) -> (w573:string[])
          n174 = Build Array(w567, "g" ("입력단위")) -> (w570:string[])
          n175 = Greater Or Equal?(x=w579, y=0.01) -> (x >= y?=w577:bool)
          n176 = Less Or Equal?(x=w586, y=w587) -> (x <= y?=w585:bool)
          n177 = Select(t=w564, s=w577, f=w565) -> (s? t:f=w576:string)
        }
        n178 = call "Unit Conversion.vi"("환산단위"="g", "입력단위"=w483, "입력값"=w485) -> ("환산값 (string)"=w484:string)  [unwired: 3 in, 5 out]
        n179 = Index Array(array=w475, index (col) #1=13 ("비활성화된 인덱스 (열)"), index (col) #2=4 ("비활성화된 인덱스 (열)")) -> (element #1=w480:string[], element #2=w478:string[])  [unwired: 2 in]
        n180 = Search 1D Array(1D array=w480, element=w484) -> (index of element=w474:i32)  [unwired: 1 in]
        n181 = Search 1D Array(1D array=w478, element=w527) -> (index of element=w502:i32)  [unwired: 1 in]
        n182 = Index Array(array=w475, index (row) #1=w474, index (col) #1=3 ("비활성화된 인덱스 (열)"), index (row) #4=w474, index (col) #4=w509, index (row) #6=w474, index (col) #6=w506, index (row) #7=w474, index (col) #7=w504, index (row) #8=w474, index (col) #8=w501, index (row) #9=w502, index (col) #9=w509, index (row) #11=w502, index (col) #11=w506, index (row) #12=w502, index (col) #12=w504, index (row) #13=w502, index (col) #13=w501) -> (element #1=w517:string, element #2=w516:string, element #3=w515:string, element #4=w514:string, element #5=w513:string, element #6=w512:string, element #7=w511:string, element #8=w510:string, element #9=w508:string, element #10=w507:string, element #11=w505:string, element #12=w503:string, element #13=w500:string)  [unwired: 8 in]
        n183 = call "Unit Conversion.vi"("환산단위"=w520, "입력단위"=w513, "입력값"=w514) -> ("환산값 (string)"=w528:string)  [unwired: 3 in, 5 out]
        n184 = call "Unit Conversion.vi"("환산단위"=w519, "입력단위"=w510, "입력값"=w511) -> ("환산값 (string)"=w522:string)  [unwired: 3 in, 5 out]
        n185 = call "Unit Conversion.vi"("환산단위"=w520, "입력단위"=w507, "입력값"=w508) -> ("환산값 (string)"=w526:string)  [unwired: 3 in, 5 out]
        n186 = call "Unit Conversion.vi"("환산단위"=w519, "입력단위"=w500, "입력값"=w503) -> ("환산값 (string)"=w521:string)  [unwired: 3 in, 5 out]
        n187 = Less Than 0?(x=w474) -> (x < 0?=w473:bool)
        n188 = Build Array(w517, w516, w515, w528, w512, w522, w527, w526, w505, w521) -> (w472:string[])
        n189 = Select(t=string[] [], s=w473, f=w472) -> (s? t:f=w471:string[])
      }
      n190 = call "Variables Data IO.vi"("Write blank data ?(F)"=w459, "Select"=Cmd_Var_Data_IO."Resolution", "error in"=w465, "Data In"=w462, "Func_ext"=w458) -> ("error out"=w464:errorcluster, "Func_ext Out"=w461:string)  [unwired: 4 in, 1 out]
      n191 = call "Variables Data IO.vi"("Write blank data ?(F)"=w459, "Select"=Cmd_Var_Data_IO."STD2", "error in"=w464, "Data In"=w467, "Func_ext"=w461) -> ("error out"=w466:errorcluster)  [unwired: 4 in, 2 out]
    }
    frame "Pressure_1", "Pressure_2", "Pressure_3" {
      n192 = case shown="\"20409-0\"" w593 {
        selector: w593 -> [_ w628 w694 w766 w839 w938 w1002 w1062 w1072]
        tunnel: [string[][] [] ("STD Data") w631 w725 w771 w850 w933 w1001 w1055 w1075] -> w599
        tunnel: [string[][] [] ("Data Out") w620 w724 w772 w849 w932 w1000 w1054 w1074] -> w592
        tunnel: w598 -> [w617 w633 w723 w774 w852 w943 w1006 w1064 w1079]
        tunnel: w597 -> [_ w634 w721 w775 w853 w944 w1007 w1065 w1080]
        tunnel: [w617 w632 w716 w773 w840 w942 w1005 w1063 w1078] -> w596
        tunnel: w595 -> [_ w627 w705 w770 w847 w939 w994 w1060 w1070]
        tunnel: w594 -> [_ w635 w703 w776 w848 w940 w1003 w1061 w1071]
        tunnel: w589 -> [_ _ _ _ _ _ _ _ w1077]
        frame Default {
        }
        frame "20406-0" {
          w638 = TRUE ("Write blank data ?(T)")
          n193 = for {
            tunnel: w635 -> [w671] mode=indexing
            tunnel: [w669] -> w629 mode=indexing
            tunnel: [w668] -> w636 mode=indexing
            n194 = Index Array(array=w671) -> (element=w673:string)  [unwired: 1 in]
            n195 = Search and Replace String(input string=w673, search string="-" ("검색 문자열")) -> (result string=w670:string, offset past replacement=w668:i32)  [unwired: 6 in, 2 out]
            n196 = Replace Array Subset(array=w671, new element=w670) -> (w669:string[])  [unwired: 1 in]
          }
          n197 = call "Match_Pressure STD.vi"("abs?(F)"=TRUE, "분류코드"=w628, "Cal STD 입력"=w627, "Condition in"=w629) -> ("Cal STD(-)"=w623:string[], "Dead Weight"=w622:string[][], "Cal STD(+)"=w621:string[], "Condition out"=w624:string[][], "단위"=w626:string, "STD Name"=w625:string)  [unwired: 2 out]
          n198 = call "Variables Data IO.vi"("Select"=Cmd_Var_Data_IO."Resolution", "error in"=w633, "Func_ext"=w634) -> ("error out"=w643:errorcluster, "Data Out"=w651:string[][], "Func_ext Out"=w640:string)  [unwired: 6 in]
          n199 = case shown="\"Pressure Balance\"" w625 {
            tunnel: [w680 w685] -> w631
            tunnel: [w679 w684] -> w637
            tunnel: w651 -> [w675 w683]
            tunnel: w624 -> [w681 w689]
            tunnel: w621 -> [w682 w688]
            tunnel: w622 -> [w674 _]
            tunnel: [w678 _] -> w645
            tunnel: [w677 _] -> w646
            tunnel: [w676 _] -> w641
            tunnel: w626 -> [_ w687]
            tunnel: w623 -> [_ w686]
            frame "Pressure Balance" {
              n200 = call "Calcu_STD Pressure_PB.vi"("Resolution"=w675, "Dead Weight"=w674, "Cal STD"=w682, "Condition"=w681) -> ("Mass set"=w677:string[][], "Uncertainty"=w678:string[][], "Data Out"=w679:string[][], "Weight set"=w676:string[][], "STD Data"=w680:string[][])  [unwired: 2 in, 1 out]
            }
            frame Default {
              # "Pre"
              n201 = call "Calcu_STD Pressure_PC.vi"("Resolution"=w683, "STD 단위"=w687, "Cal STD (-)"=w686, "Cal STD (+)"=w688, "Condition"=w689) -> ("Data Out"=w684:string[][], "STD Data"=w685:string[][])  [unwired: 4 in, 1 out]
            }
          }
          n202 = call "Variables Data IO.vi"("Write blank data ?(F)"=w638, "Select"=Cmd_Var_Data_IO."Condition_Temp", "error in"=w643, "Data In"=w641, "Func_ext"=w640) -> ("error out"=w642:errorcluster, "Func_ext Out"=w639:string)  [unwired: 4 in, 1 out]
          n203 = call "Variables Data IO.vi"("Write blank data ?(F)"=w638, "Select"=Cmd_Var_Data_IO."STD2", "error in"=w642, "Data In"=w646, "Func_ext"=w639) -> ("error out"=w648:errorcluster, "Func_ext Out"=w647:string)  [unwired: 4 in, 1 out]
          n204 = call "Variables Data IO.vi"("Write blank data ?(F)"=w638, "Select"=Cmd_Var_Data_IO."STD3", "error in"=w648, "Data In"=w645, "Func_ext"=w647) -> ("error out"=w632:errorcluster)  [unwired: 4 in, 2 out]
          n205 = for {
            tunnel: w637 -> [w654] mode=indexing
            tunnel: w636 -> [w655] mode=indexing
            tunnel: [w653] -> w620 mode=indexing
            n206 = case shown="기본" w655 {
              tunnel: w654 -> [w662 w667]
              tunnel: [w658 w667] -> w653
              frame Default {
                w665 = "-" ("문자열")
                w656 = 4 ("인덱스")
                w657 = 1 ("인덱스")
                n207 = Index Array(array=w662, index #1=w657, index #3=w656) -> (element #1=w666:string, element #2=w664:string, element #3=w663:string)  [unwired: 1 in]
                n208 = Concatenate Strings(w665, w666) -> (w661:string)
                n209 = Concatenate Strings(w665, w664) -> (w660:string)
                n210 = Concatenate Strings(w665, w663) -> (w659:string)
                n211 = Replace Array Subset(array=w662, new element #1=w661, index #1=w657, new element #2=w660, new element #3=w659, index #3=w656) -> (w658:string[])  [unwired: 1 in]
              }
              frame -1 {
              }
            }
          }
        }
        frame "20408-0", "20411-1", "20411-4" {
          w706 = TRUE ("Write blank data ?(T)")
          n212 = call "Match_Pressure STD.vi"("분류코드"=w694, "Cal STD 입력"=w705, "Condition in"=w703) -> ("Cal STD(-)"=w692:string[], "Dead Weight"=w691:string[][], "Cal STD(+)"=w690:string[], "Condition out"=w693:string[][], "단위"=w704:string, "STD Name"=w697:string)  [unwired: 1 in, 2 out]
          n213 = Index Array(array=w703, index (col)=0 ("비활성화된 인덱스 (열)")) -> (element=w701:string[])  [unwired: 1 in]
          n214 = Fract/Exp String To Number(string=w701) -> (number=w700:dbl[])  [unwired: 3 in, 1 out]
          n215 = Array Max & Min(array=w700) -> (max value=w699:dbl)  [unwired: 3 out]
          n216 = Less Or Equal To 0?(x=w699) -> (x <= 0?=w698:bool)
          n217 = call "Variables Data IO.vi"("Select"=Cmd_Var_Data_IO."Resolution", "error in"=w723, "Func_ext"=w721) -> ("error out"=w711:errorcluster, "Data Out"=w720:string[][], "Func_ext Out"=w708:string)  [unwired: 6 in]
          n218 = Select(t="Pressure Calibrator", s=w698, f=w697) -> (s? t:f=w696:string)
          n219 = case shown="\"Pressure Balance\"" w696 {
            tunnel: [w728 w744] -> w725
            tunnel: [w727 w745] -> w724
            tunnel: w720 -> [w726 w735]
            tunnel: w690 -> [w732 w748]
            tunnel: w691 -> [_ w734]
            tunnel: [_ w738] -> w713
            tunnel: [_ w737] -> w714
            tunnel: [_ w736] -> w709
            tunnel: w692 -> [w731 w747]
            tunnel: w704 -> [w730 _]
            tunnel: w693 -> [w729 w743]
            frame Default {
              # "Pressure Calibrator"
              n220 = call "Calcu_STD Pressure_PC.vi"("Resolution"=w726, "STD 단위"=w730, "Cal STD (-)"=w731, "Cal STD (+)"=w732, "Condition"=w729) -> ("Data Out"=w727:string[][], "STD Data"=w728:string[][])  [unwired: 4 in, 1 out]
            }
            frame "Pressure Balance" {
              # "Pressure Balance"
              n221 = call "Calcu_STD Pressure_PC.vi"("Resolution"=w735, "STD 단위"="MPa", "Cal STD (-)"=w747, "Condition"=w743) -> ("Data Out"=w740:string[][], "STD Data"=w742:string[][])  [unwired: 5 in, 1 out]
              n222 = call "Calcu_STD Pressure_PB.vi"("Resolution"=w735, "Dead Weight"=w734, "Cal STD"=w748, "Condition"=w743) -> ("Mass set"=w737:string[][], "Uncertainty"=w738:string[][], "Data Out"=w739:string[][], "Weight set"=w736:string[][], "STD Data"=w741:string[][])  [unwired: 2 in, 1 out]
              n223 = Fract/Exp String To Number(string=w743) -> (number=w746:dbl[][])  [unwired: 3 in, 1 out]
              n224 = for {
                tunnel: w746 -> [w757] mode=indexing
                tunnel: w742 -> [w754] mode=indexing
                tunnel: w741 -> [w753] mode=indexing
                tunnel: w740 -> [w752] mode=indexing
                tunnel: w739 -> [w751] mode=indexing
                tunnel: [w750] -> w745 mode=indexing
                tunnel: [w749] -> w744 mode=indexing
                n225 = Index Array(array=w757) -> (element=w756:dbl)  [unwired: 1 in]
                n226 = Less Than 0?(x=w756) -> (x < 0?=w755:bool)
                n227 = case shown="참" w755 {
                  tunnel: w754 -> [_ w761]
                  tunnel: w753 -> [w759 _]
                  tunnel: [w759 w761] -> w749
                  tunnel: w752 -> [_ w760]
                  tunnel: [w758 w760] -> w750
                  tunnel: w751 -> [w758 _]
                  frame False {
                  }
                  frame True {
                  }
                }
              }
            }
          }
          n228 = call "Variables Data IO.vi"("Write blank data ?(F)"=w706, "Select"=Cmd_Var_Data_IO."Condition_Temp", "error in"=w711, "Data In"=w709, "Func_ext"=w708) -> ("error out"=w710:errorcluster, "Func_ext Out"=w707:string)  [unwired: 4 in, 1 out]
          n229 = call "Variables Data IO.vi"("Write blank data ?(F)"=w706, "Select"=Cmd_Var_Data_IO."STD2", "error in"=w710, "Data In"=w714, "Func_ext"=w707) -> ("error out"=w717:errorcluster, "Func_ext Out"=w715:string)  [unwired: 4 in, 1 out]
          n230 = call "Variables Data IO.vi"("Write blank data ?(F)"=w706, "Select"=Cmd_Var_Data_IO."STD3", "error in"=w717, "Data In"=w713, "Func_ext"=w715) -> ("error out"=w716:errorcluster)  [unwired: 4 in, 2 out]
        }
        frame "20409-0" {
          w779 = TRUE ("Write blank data ?(T)")
          n231 = for {
            tunnel: w776 -> [w812] mode=indexing
            tunnel: [w810] -> w769 mode=indexing
            tunnel: [w809] -> w777 mode=indexing
            n232 = Index Array(array=w812) -> (element=w814:string)  [unwired: 1 in]
            n233 = Search and Replace String(input string=w814, search string="-" ("검색 문자열")) -> (result string=w811:string, offset past replacement=w809:i32)  [unwired: 6 in, 2 out]
            n234 = Replace Array Subset(array=w812, new element=w811) -> (w810:string[])  [unwired: 1 in]
          }
          n235 = call "Variables Data IO.vi"("Select"=Cmd_Var_Data_IO."Resolution", "error in"=w774, "Func_ext"=w775) -> ("error out"=w784:errorcluster, "Data Out"=w792:string[][], "Func_ext Out"=w781:string)  [unwired: 6 in]
          n236 = call "Match_Pressure STD.vi"("분류코드"=w766, "Cal STD 입력"=w770, "Condition in"=w769) -> ("Cal STD(-)"=w764:string[], "Dead Weight"=w762:string[][], "Cal STD(+)"=w763:string[], "Condition out"=w765:string[][], "단위"=w767:string, "STD Name"=w768:string)  [unwired: 1 in, 2 out]
          n237 = case shown="\"Pressure Balance\"" w768 {
            tunnel: [w821 w826] -> w771
            tunnel: [w820 w825] -> w778
            tunnel: w792 -> [w816 w824]
            tunnel: w765 -> [w822 w830]
            tunnel: w763 -> [w823 w829]
            tunnel: w762 -> [w815 _]
            tunnel: [w819 _] -> w786
            tunnel: [w818 _] -> w787
            tunnel: [w817 _] -> w782
            tunnel: w767 -> [_ w828]
            tunnel: w764 -> [_ w827]
            frame "Pressure Balance" {
              n238 = call "Calcu_STD Pressure_PB.vi"("Resolution"=w816, "Dead Weight"=w815, "Cal STD"=w823, "Condition"=w822) -> ("Mass set"=w818:string[][], "Uncertainty"=w819:string[][], "Data Out"=w820:string[][], "Weight set"=w817:string[][], "STD Data"=w821:string[][])  [unwired: 2 in, 1 out]
            }
            frame Default {
              # "Pre"
              n239 = call "Calcu_STD Pressure_PC.vi"("Resolution"=w824, "STD 단위"=w828, "Cal STD (-)"=w827, "Cal STD (+)"=w829, "Condition"=w830) -> ("Data Out"=w825:string[][], "STD Data"=w826:string[][])  [unwired: 4 in, 1 out]
            }
          }
          n240 = call "Variables Data IO.vi"("Write blank data ?(F)"=w779, "Select"=Cmd_Var_Data_IO."Condition_Temp", "error in"=w784, "Data In"=w782, "Func_ext"=w781) -> ("error out"=w783:errorcluster, "Func_ext Out"=w780:string)  [unwired: 4 in, 1 out]
          n241 = call "Variables Data IO.vi"("Write blank data ?(F)"=w779, "Select"=Cmd_Var_Data_IO."STD2", "error in"=w783, "Data In"=w787, "Func_ext"=w780) -> ("error out"=w789:errorcluster, "Func_ext Out"=w788:string)  [unwired: 4 in, 1 out]
          n242 = call "Variables Data IO.vi"("Write blank data ?(F)"=w779, "Select"=Cmd_Var_Data_IO."STD3", "error in"=w789, "Data In"=w786, "Func_ext"=w788) -> ("error out"=w773:errorcluster)  [unwired: 4 in, 2 out]
          n243 = for {
            tunnel: w778 -> [w795] mode=indexing
            tunnel: w777 -> [w796] mode=indexing
            tunnel: [w794] -> w772 mode=indexing
            n244 = case shown="기본" w796 {
              tunnel: w795 -> [w803 w808]
              tunnel: [w799 w808] -> w794
              frame Default {
                w806 = "-" ("문자열")
                w797 = 4 ("인덱스")
                w798 = 1 ("인덱스")
                n245 = Index Array(array=w803, index #1=w798, index #3=w797) -> (element #1=w807:string, element #2=w805:string, element #3=w804:string)  [unwired: 1 in]
                n246 = Concatenate Strings(w806, w807) -> (w802:string)
                n247 = Concatenate Strings(w806, w805) -> (w801:string)
                n248 = Concatenate Strings(w806, w804) -> (w800:string)
                n249 = Replace Array Subset(array=w803, new element #1=w802, index #1=w798, new element #2=w801, new element #3=w800, index #3=w797) -> (w799:string[])  [unwired: 1 in]
              }
              frame -1 {
              }
            }
          }
        }
        frame "20412-1" {
          w854 = TRUE ("Write blank data ?(T)")
          n250 = call "Match_Pressure STD.vi"("분류코드"=w839, "Cal STD 입력"=w847, "Condition in"=w848) -> ("Cal STD(-)"=w837:string[], "Dead Weight"=w835:string[][], "Cal STD(+)"=w836:string[], "Condition out"=w838:string[][], "Cal STD(DMM)"=w834:string[][], "단위"=w845:string, "Power Supply?"=w832:string, "STD Name"=w846:string)  [unwired: 1 in]
          n251 = call "Variables Data IO.vi"("Select"=Cmd_Var_Data_IO."Resolution", "error in"=w852, "Func_ext"=w853) -> ("error out"=w857:errorcluster, "Data Out"=w865:string[][], "Func_ext Out"=w855:string)  [unwired: 6 in]
          n252 = case shown="기본" w846 {
            tunnel: [w916 w922] -> w850
            tunnel: [w915 w921] -> w849
            tunnel: w865 -> [w910 w919]
            tunnel: w838 -> [w917 w926]
            tunnel: w836 -> [w918 w925]
            tunnel: w835 -> [w909 _]
            tunnel: [w914 _] -> w859
            tunnel: [w913 _] -> w860
            tunnel: [w911 _] -> w856
            tunnel: w845 -> [_ w924]
            tunnel: [w912 w920] -> w833
            tunnel: w837 -> [_ w923]
            frame "Pressure Balance" {
              n253 = call "Calcu_STD Pressure_PB.vi"("Resolution"=w910, "Dead Weight"=w909, "Cal STD"=w918, "Condition"=w917) -> ("배열"=w912:dbl[], "Mass set"=w913:string[][], "Uncertainty"=w914:string[][], "Data Out"=w915:string[][], "Weight set"=w911:string[][], "STD Data"=w916:string[][])  [unwired: 2 in]
            }
            frame Default {
              # "Pre"
              n254 = call "Calcu_STD Pressure_PC.vi"("Resolution"=w919, "STD 단위"=w924, "Cal STD (-)"=w923, "Cal STD (+)"=w925, "Condition"=w926) -> ("배열"=w920:dbl[], "Data Out"=w921:string[][], "STD Data"=w922:string[][])  [unwired: 4 in]
            }
          }
          n255 = call "Variables Data IO.vi"("Write blank data ?(F)"=w854, "Select"=Cmd_Var_Data_IO."Condition_Temp", "error in"=w857, "Data In"=w856, "Func_ext"=w855) -> ("error out"=w844:errorcluster, "Func_ext Out"=w843:string)  [unwired: 4 in, 1 out]
          n256 = for {
            tunnel: [w870] -> w831 mode=indexing
            tunnel: w834 -> [w869]
            tunnel: w833 -> [w868] mode=indexing
            tunnel: w832 -> [w867]
            n257 = for {
              tunnel: [w902] -> w870
              tunnel: w869 -> [w900] mode=indexing
              tunnel: w868 -> [w888]
              tunnel: w867 -> [w882]
              stop <- w907 stop-if-true
              n258 = Index Array(array=w900, index #1=11 ("인덱스"), index #2=1 ("비활성화된 인덱스 (열)"), index #3=12 ("비활성화된 인덱스 (열)"), index #5=15 ("인덱스"), index #9=19 ("인덱스"), index #10=21 ("인덱스"), index #11=24 ("인덱스")) -> (element #1=w872:string, element #2=w871:string, element #3=w879:string, element #4=w887:string, element #5=w885:string, element #6=w884:string, element #7=w890:string, element #8=w889:string, element #9=w905:string, element #10=w899:string, element #11=w877:string, element #12=w876:string, element #13=w875:string, element #14=w874:string)  [unwired: 7 in]
              n259 = Fract/Exp String To Number(string=w872) -> (number=w908:dbl)  [unwired: 3 in, 1 out]
              n260 = Less?(x=w888, y=w908) -> (x < y?=w907:bool)
              n261 = call "Unit Conversion.vi"("환산단위"=w879, "입력단위"=w884, "입력값"=w887) -> ("환산값 (string)"=w891:string)  [unwired: 3 in, 5 out]
              n262 = call "Unit Conversion.vi"("환산단위"=w879, "입력단위"=w884, "입력값"=w885) -> ("환산값 (string)"=w883:string)  [unwired: 3 in, 5 out]
              n263 = call "Unit Conversion.vi"("환산단위"=w879, "입력단위"=w889, "입력값"=w890) -> ("환산단위"=w893:string, "환산값 (string)"=w892:string)  [unwired: 3 in, 4 out]
              n264 = call "Unit Conversion.vi"("환산단위"=w879, "입력단위"=w899, "입력값"=w905) -> ("환산단위"=w901:string, "환산값 (string)"=w903:string)  [unwired: 3 in, 4 out]
              n265 = call "Unit Conversion.vi"("환산단위"="실수", "입력단위"=w876, "입력값"=w877) -> ("환산단위"=w894:string, "환산값 (string)"=w895:string)  [unwired: 3 in, 4 out]
              n266 = call "Unit Conversion.vi"("환산단위"=w879, "입력단위"=w874, "입력값"=w875) -> ("환산단위"=w897:string, "환산값 (string)"=w898:string)  [unwired: 3 in, 4 out]
              n267 = Build Array(w871, w891, w883, w892, w893, w903, w901, w895, w894, w898, w897, w882) -> (w902:string[])
            }
          }
          n268 = call "Variables Data IO.vi"("Select"=Cmd_Var_Data_IO."STD4", "error in"=w844, "Data In"=w831, "Func_ext"=w843) -> ("error out"=w841:errorcluster, "Func_ext Out"=w842:string)  [unwired: 5 in, 1 out]
          n269 = call "Variables Data IO.vi"("Write blank data ?(F)"=w854, "Select"=Cmd_Var_Data_IO."STD2", "error in"=w841, "Data In"=w860, "Func_ext"=w842) -> ("error out"=w862:errorcluster, "Func_ext Out"=w861:string)  [unwired: 4 in, 1 out]
          n270 = call "Variables Data IO.vi"("Write blank data ?(F)"=w854, "Select"=Cmd_Var_Data_IO."STD3", "error in"=w862, "Data In"=w859, "Func_ext"=w861) -> ("error out"=w840:errorcluster)  [unwired: 4 in, 2 out]
        }
        frame "20412-2" {
          n271 = call "Match_Pressure STD.vi"("abs?(F)"=TRUE, "분류코드"=w938, "Cal STD 입력"=w939, "Condition in"=w940) -> ("Cal STD(+)"=w934:string[], "Condition out"=w935:string[][], "Cal STD(DMM)"=w930:string[][], "단위"=w936:string, "Power Supply?"=w929:string)  [unwired: 3 out]
          n272 = call "Variables Data IO.vi"("Select"=Cmd_Var_Data_IO."Resolution", "error in"=w943, "Func_ext"=w944) -> ("error out"=w946:errorcluster, "Data Out"=w927:string[][], "Func_ext Out"=w945:string)  [unwired: 6 in]
          n273 = call "Calcu_STD Pressure_PC.vi"("Resolution"=w927, "STD 단위"=w936, "Cal STD (+)"=w934, "Condition"=w935) -> ("배열"=w931:dbl[], "Data Out"=w932:string[][], "STD Data"=w933:string[][])  [unwired: 5 in]
          n274 = for {
            tunnel: [w951] -> w928 mode=indexing
            tunnel: w930 -> [w950]
            tunnel: w931 -> [w949] mode=indexing
            tunnel: w929 -> [w948]
            n275 = for {
              tunnel: [w983] -> w951
              tunnel: w950 -> [w981] mode=indexing
              tunnel: w949 -> [w969]
              tunnel: w948 -> [w963]
              stop <- w988 stop-if-true
              n276 = Index Array(array=w981, index #1=11 ("인덱스"), index #2=1 ("비활성화된 인덱스 (열)"), index #3=12 ("비활성화된 인덱스 (열)"), index #5=15 ("인덱스"), index #9=19 ("인덱스"), index #10=21 ("인덱스"), index #11=24 ("인덱스")) -> (element #1=w953:string, element #2=w952:string, element #3=w960:string, element #4=w968:string, element #5=w966:string, element #6=w965:string, element #7=w971:string, element #8=w970:string, element #9=w986:string, element #10=w980:string, element #11=w958:string, element #12=w957:string, element #13=w956:string, element #14=w955:string)  [unwired: 7 in]
              n277 = Fract/Exp String To Number(string=w953) -> (number=w989:dbl)  [unwired: 3 in, 1 out]
              n278 = Less?(x=w969, y=w989) -> (x < y?=w988:bool)
              n279 = call "Unit Conversion.vi"("환산단위"=w960, "입력단위"=w965, "입력값"=w968) -> ("환산값 (string)"=w972:string)  [unwired: 3 in, 5 out]
              n280 = call "Unit Conversion.vi"("환산단위"=w960, "입력단위"=w965, "입력값"=w966) -> ("환산값 (string)"=w964:string)  [unwired: 3 in, 5 out]
              n281 = call "Unit Conversion.vi"("환산단위"=w960, "입력단위"=w970, "입력값"=w971) -> ("환산단위"=w974:string, "환산값 (string)"=w973:string)  [unwired: 3 in, 4 out]
              n282 = call "Unit Conversion.vi"("환산단위"=w960, "입력단위"=w980, "입력값"=w986) -> ("환산단위"=w982:string, "환산값 (string)"=w984:string)  [unwired: 3 in, 4 out]
              n283 = call "Unit Conversion.vi"("환산단위"="실수", "입력단위"=w957, "입력값"=w958) -> ("환산단위"=w975:string, "환산값 (string)"=w976:string)  [unwired: 3 in, 4 out]
              n284 = call "Unit Conversion.vi"("환산단위"=w960, "입력단위"=w955, "입력값"=w956) -> ("환산단위"=w978:string, "환산값 (string)"=w979:string)  [unwired: 3 in, 4 out]
              n285 = Build Array(w952, w972, w964, w973, w974, w984, w982, w976, w975, w979, w978, w963) -> (w983:string[])
            }
          }
          n286 = call "Variables Data IO.vi"("Select"=Cmd_Var_Data_IO."STD4", "error in"=w946, "Data In"=w928, "Func_ext"=w945) -> ("error out"=w942:errorcluster)  [unwired: 5 in, 2 out]
        }
        frame "20412-3" {
          n287 = call "Match_Pressure STD.vi"("분류코드"=w1002, "Cal STD 입력"=w994, "Condition in"=w1003) -> ("Cal STD(-)"=w990:string[], "Cal STD(+)"=w991:string[], "Condition out"=w992:string[][], "Cal STD(DMM)"=w998:string[][], "단위"=w993:string, "Power Supply?"=w997:string)  [unwired: 1 in, 2 out]
          n288 = call "Variables Data IO.vi"("Select"=Cmd_Var_Data_IO."Resolution", "error in"=w1006, "Func_ext"=w1007) -> ("error out"=w1009:errorcluster, "Data Out"=w995:string[][], "Func_ext Out"=w1008:string)  [unwired: 6 in]
          n289 = call "Calcu_STD Pressure_PC.vi"("Resolution"=w995, "STD 단위"=w993, "Cal STD (-)"=w990, "Cal STD (+)"=w991, "Condition"=w992) -> ("배열"=w999:dbl[], "Data Out"=w1000:string[][], "STD Data"=w1001:string[][])  [unwired: 4 in]
          n290 = for {
            tunnel: [w1014] -> w996 mode=indexing
            tunnel: w998 -> [w1013]
            tunnel: w999 -> [w1012] mode=indexing
            tunnel: w997 -> [w1011]
            n291 = for {
              tunnel: [w1046] -> w1014
              tunnel: w1013 -> [w1044] mode=indexing
              tunnel: w1012 -> [w1032]
              tunnel: w1011 -> [w1026]
              stop <- w1051 stop-if-true
              n292 = Index Array(array=w1044, index #1=11 ("인덱스"), index #2=1 ("비활성화된 인덱스 (열)"), index #3=12 ("비활성화된 인덱스 (열)"), index #5=15 ("인덱스"), index #9=19 ("인덱스"), index #10=21 ("인덱스"), index #11=24 ("인덱스")) -> (element #1=w1016:string, element #2=w1015:string, element #3=w1023:string, element #4=w1031:string, element #5=w1029:string, element #6=w1028:string, element #7=w1034:string, element #8=w1033:string, element #9=w1049:string, element #10=w1043:string, element #11=w1021:string, element #12=w1020:string, element #13=w1019:string, element #14=w1018:string)  [unwired: 7 in]
              n293 = Fract/Exp String To Number(string=w1016) -> (number=w1052:dbl)  [unwired: 3 in, 1 out]
              n294 = Less?(x=w1032, y=w1052) -> (x < y?=w1051:bool)
              n295 = call "Unit Conversion.vi"("환산단위"=w1023, "입력단위"=w1028, "입력값"=w1031) -> ("환산값 (string)"=w1035:string)  [unwired: 3 in, 5 out]
              n296 = call "Unit Conversion.vi"("환산단위"=w1023, "입력단위"=w1028, "입력값"=w1029) -> ("환산값 (string)"=w1027:string)  [unwired: 3 in, 5 out]
              n297 = call "Unit Conversion.vi"("환산단위"=w1023, "입력단위"=w1033, "입력값"=w1034) -> ("환산단위"=w1037:string, "환산값 (string)"=w1036:string)  [unwired: 3 in, 4 out]
              n298 = call "Unit Conversion.vi"("환산단위"=w1023, "입력단위"=w1043, "입력값"=w1049) -> ("환산단위"=w1045:string, "환산값 (string)"=w1047:string)  [unwired: 3 in, 4 out]
              n299 = call "Unit Conversion.vi"("환산단위"="실수", "입력단위"=w1020, "입력값"=w1021) -> ("환산단위"=w1038:string, "환산값 (string)"=w1039:string)  [unwired: 3 in, 4 out]
              n300 = call "Unit Conversion.vi"("환산단위"=w1023, "입력단위"=w1018, "입력값"=w1019) -> ("환산단위"=w1041:string, "환산값 (string)"=w1042:string)  [unwired: 3 in, 4 out]
              n301 = Build Array(w1015, w1035, w1027, w1036, w1037, w1047, w1045, w1039, w1038, w1042, w1041, w1026) -> (w1046:string[])
            }
          }
          n302 = call "Variables Data IO.vi"("Select"=Cmd_Var_Data_IO."STD4", "error in"=w1009, "Data In"=w996, "Func_ext"=w1008) -> ("error out"=w1005:errorcluster)  [unwired: 5 in, 2 out]
        }
        frame "20413-0" {
          n303 = call "Match_Pressure STD.vi"("분류코드"=w1062, "Cal STD 입력"=w1060, "Condition in"=w1061) -> ("Cal STD(-)"=w1057:string[], "Cal STD(+)"=w1056:string[], "Condition out"=w1058:string[][], "단위"=w1059:string)  [unwired: 1 in, 4 out]
          n304 = call "Variables Data IO.vi"("Select"=Cmd_Var_Data_IO."Resolution", "error in"=w1064, "Func_ext"=w1065) -> ("error out"=w1063:errorcluster, "Data Out"=w1053:string[][])  [unwired: 6 in, 1 out]
          n305 = call "Calcu_STD Pressure_PC.vi"("Resolution"=w1053, "STD 단위"=w1059, "Cal STD (-)"=w1057, "Cal STD (+)"=w1056, "Condition"=w1058) -> ("Data Out"=w1054:string[][], "STD Data"=w1055:string[][])  [unwired: 4 in, 1 out]
        }
        frame "20414-0" {
          n306 = call "Match_Pressure STD.vi"("분류코드"=w1072, "Cal STD 입력"=w1070, "Condition in"=w1071) -> ("Cal STD(+)"=w1069:string[], "Condition out"=w1067:string[][], "단위"=w1068:string)  [unwired: 1 in, 5 out]
          n307 = Index Array(array=w1077) -> (element=w1076:string[])  [unwired: 2 in]
          n308 = call "Variables Data IO.vi"("Select"=Cmd_Var_Data_IO."Resolution", "error in"=w1079, "Func_ext"=w1080) -> ("error out"=w1078:errorcluster, "Data Out"=w1073:string[][])  [unwired: 6 in, 1 out]
          n309 = call "Calcu_STD Pressure_PC.vi"("Resolution"=w1073, "STD 단위"=w1068, "Cal STD (-)"=w1076, "Cal STD (+)"=w1069, "Condition"=w1067) -> ("Data Out"=w1074:string[][], "STD Data"=w1075:string[][])  [unwired: 4 in, 1 out]
        }
      }
      n310 = case shown="\"Pressure_2\"" w590 {
        tunnel: w592 -> [w601 w610]
        tunnel: [w600 w609] -> w591
        frame Default {
          n311 = for {
            tunnel: w601 -> [w608] mode=indexing
            tunnel: [w604] -> w600 mode=indexing
            n312 = Index Array(array=w608, index #1=1 ("인덱스"), index #2=3 ("인덱스")) -> (element #1=w606:string, element #2=w605:string)
            n313 = Format Into String(format string="%s %s" ("포맷 문자열"), w606, w605) -> (resulting string=w604:string)  [unwired: 2 in, 1 out]
          }
        }
        frame "Pressure_2" {
          n314 = for {
            tunnel: w610 -> [w616] mode=indexing
            tunnel: [w612] -> w609 mode=indexing
            n315 = Index Array(array=w616, index #1=4 ("인덱스")) -> (element #1=w614:string, element #2=w613:string)  [unwired: 1 in]
            n316 = Format Into String(format string="%s %s" ("포맷 문자열"), w614, w613) -> (resulting string=w612:string)  [unwired: 2 in, 1 out]
          }
        }
      }
    }
    frame "Pressure_4" {
      n317 = call-poly "Data Classification.vi"("인덱스"=2, "DATA 입력"=w1088, "검색 문자열"="Pressure Logger(abs)") -> ("DATA 출력"=w1086:string[][])  [unwired: 4 in, 4 out]
      n318 = Index Array(array=w1086) -> (element=w1084:string[])  [unwired: 2 in]
      n319 = for {
        tunnel: w1085 -> [_] mode=indexing
        tunnel: w1084 -> [w1090]
        tunnel: [w1090] -> w1083 mode=indexing
      }
    }
    frame "Resistance Meter" {
      n320 = case shown="\"Resistance Meter\", 기본" w1091 {
        tunnel: ["Resistance Source"] -> w1095
        tunnel: ["kΩ" ("환산단위")] -> w1094
        frame "Resistance Meter", Default {
        }
      }
      n321 = call-poly "Data Classification.vi"("인덱스"=2, "DATA 입력"=w1102, "검색 문자열"=w1095) -> ("DATA 출력"=w1097:string[][])  [unwired: 4 in, 4 out]
      n322 = for {
        tunnel: w1097 -> [w1183] mode=indexing
        tunnel: [w1178] -> w1096 mode=indexing
        tunnel: w1094 -> [w1173]
        n323 = Index Array(array=w1183, index #1=13 ("인덱스")) -> (element #1=w1184:string, element #2=w1182:string, element #3=w1180:string, element #4=w1181:string)  [unwired: 3 in]
        n324 = call "Unit Conversion.vi"("환산단위"=w1173, "입력단위"=w1181, "입력값"=w1184) -> ("환산값 (string)"=w1177:string)  [unwired: 3 in, 5 out]
        n325 = call "Unit Conversion.vi"("환산단위"=w1173, "입력단위"=w1181, "입력값"=w1182) -> ("환산값 (string)"=w1176:string)  [unwired: 3 in, 5 out]
        n326 = call "Unit Conversion.vi"("환산단위"=w1173, "입력단위"=w1181, "입력값"=w1180) -> ("환산단위"=w1174:string, "환산값 (string)"=w1175:string)  [unwired: 3 in, 4 out]
        n327 = Replace Array Subset(array=w1183, new element #1=w1177, index #1=13 ("인덱스"), new element #2=w1176, new element #3=w1175, new element #4=w1174) -> (w1178:string[])  [unwired: 3 in]
      }
      n328 = call-poly "Data Sorting.vi"("기준열"=u16 13, "error in (no error)"=w1101, "Data in"=w1096) -> ("error out"=w1099:errorcluster, "Data out"=w1093:string[][])  [unwired: 7 in]
      n329 = for {
        tunnel: w1093 -> [w1126]
        tunnel: w1100 -> [w1125] mode=indexing
        tunnel: [w1119] -> w1092 mode=indexing
        w1116 = 24 ("인덱스")
        w1117 = 21 ("인덱스")
        w1118 = 13 ("인덱스")
        n330 = Index Array(array=w1125) -> (element #3=w1122:string, element #4=w1124:string)  [unwired: 4 in, 2 out]
        n331 = Fract/Exp String To Number(string=w1122) -> (number=w1123:dbl)  [unwired: 3 in, 1 out]
        n332 = for {
          tunnel: w1126 -> [w1139] mode=indexing
          tunnel: w1124 -> [w1127]
          tunnel: [w1139] -> w1120
          tunnel: w1123 -> [w1155]
          tunnel: w1118 -> [w1138]
          tunnel: w1117 -> [w1142]
          tunnel: w1116 -> [w1141]
          tunnel: [w1140] -> w1121
          tunnel: [w1137] -> w1115
          tunnel: [w1136] -> w1114
          tunnel: [w1135] -> w1113
          tunnel: [w1134] -> w1112
          tunnel: [w1133] -> w1111
          tunnel: [w1132] -> w1110
          tunnel: [w1131] -> w1109
          tunnel: [w1130] -> w1108
          tunnel: [w1129] -> w1107
          tunnel: [w1128] -> w1106
          stop <- w1140 stop-if-true
          n333 = Index Array(array=w1139, index #1=w1138, index #8=w1142, index #9=w1141) -> (element #1=w1157:string, element #2=w1154:string, element #3=w1153:string, element #4=w1152:string, element #5=w1151:string, element #6=w1150:string, element #7=w1149:string, element #8=w1148:string, element #9=w1147:string, element #10=w1146:string, element #11=w1144:string, element #12=w1143:string)  [unwired: 9 in]
          n334 = call "Unit Conversion.vi"("환산단위"=w1127, "입력단위"=w1152, "입력값"=w1157) -> ("환산단위"=w1134:string, "환산값 (DBL)"=w1156:dbl, "환산값 (string)"=w1137:string)  [unwired: 3 in, 3 out]
          n335 = call "Unit Conversion.vi"("환산단위"=w1127, "입력단위"=w1152, "입력값"=w1154) -> ("환산값 (string)"=w1136:string)  [unwired: 3 in, 5 out]
          n336 = call "Unit Conversion.vi"("환산단위"=w1127, "입력단위"=w1152, "입력값"=w1153) -> ("환산값 (string)"=w1135:string)  [unwired: 3 in, 5 out]
          n337 = call "Unit Conversion.vi"("환산단위"=w1127, "입력단위"=w1150, "입력값"=w1151) -> ("환산값 (string)"=w1133:string)  [unwired: 3 in, 5 out]
          n338 = call "Unit Conversion.vi"("환산단위"=w1127, "입력단위"=w1148, "입력값"=w1149) -> ("환산값 (string)"=w1132:string)  [unwired: 3 in, 5 out]
          n339 = call "Unit Conversion.vi"("환산단위"="실수", "입력단위"=w1146, "입력값"=w1147) -> ("환산단위"=w1130:string, "환산값 (string)"=w1131:string)  [unwired: 3 in, 4 out]
          n340 = call "Unit Conversion.vi"("환산단위"=w1127, "입력단위"=w1143, "입력값"=w1144) -> ("환산단위"=w1128:string, "환산값 (string)"=w1129:string)  [unwired: 3 in, 4 out]
          n341 = Greater Or Equal?(x=w1156, y=w1155) -> (x >= y?=w1140:bool)
        }
        n342 = case shown="참" w1121 {
          tunnel: w1120 -> [_ w1172]
          tunnel: [_ w1171] -> w1119
          tunnel: w1118 -> [_ w1170]
          tunnel: w1115 -> [_ w1169]
          tunnel: w1114 -> [_ w1168]
          tunnel: w1113 -> [_ w1167]
          tunnel: w1112 -> [_ w1164]
          tunnel: w1111 -> [_ w1166]
          tunnel: w1110 -> [_ w1165]
          tunnel: w1109 -> [_ w1161]
          tunnel: w1117 -> [_ w1163]
          tunnel: w1108 -> [_ w1160]
          tunnel: w1116 -> [_ w1162]
          tunnel: w1107 -> [_ w1159]
          tunnel: w1106 -> [_ w1158]
          frame False {
          }
          frame True {
            n343 = Replace Array Subset(array=w1172, new element #1=w1169, index #1=w1170, new element #2=w1168, new element #3=w1167, new element #4=w1164, new element #5=w1166, new element #6=w1164, new element #7=w1165, new element #8=w1164, index #8=w1163, new element #9=w1161, index #9=w1162, new element #10=w1160, new element #11=w1159, new element #12=w1158) -> (w1171:string[])  [unwired: 9 in]
          }
        }
      }
    }
    frame "Torque_1" {
      w1215 = TRUE ("Write blank data ?(T)")
      w1220 = 0 ("비활성화된 인덱스 (열)")
      w1228 = 2 ("인덱스")
      n344 = call-poly "Data Classification.vi"("인덱스"=w1228, "DATA 입력"=w1230, "검색 문자열"="Torque Arm") -> ("DATA 출력"=w1213:string[][])  [unwired: 4 in, 4 out]
      n345 = call-poly "Data Classification.vi"("인덱스"=w1228, "DATA 입력"=w1230, "검색 문자열"="Dead Weight (Force)") -> ("DATA 출력"=w1226:string[][])  [unwired: 4 in, 4 out]
      n346 = for {
        tunnel: w1213 -> [w1253] mode=indexing
        tunnel: [w1250] -> w1212
        tunnel: [w1252] -> w1201 mode=indexing
        tunnel: [w1235] -> w1194
        tunnel: [w1234] -> w1197
        w1239 = "m" ("환산단위")
        n347 = Index Array(array=w1253, index #1=13 ("비활성화된 인덱스 (열)"), index #8=21 ("인덱스"), index #9=24 ("인덱스")) -> (element #1=w1261:string, element #2=w1259:string, element #3=w1258:string, element #4=w1257:string, element #5=w1256:string, element #6=w1255:string, element #7=w1254:string, element #8=w1244:string, element #9=w1241:string, element #10=w1240:string)  [unwired: 7 in]
        n348 = call "Unit Conversion.vi"("환산단위"=w1239, "입력단위"=w1257, "입력값"=w1261) -> ("환산값 (string)"=w1250:string)  [unwired: 3 in, 5 out]
        n349 = call "Unit Conversion.vi"("환산단위"=w1239, "입력단위"=w1257, "입력값"=w1259) -> ("환산값 (string)"=w1249:string)  [unwired: 3 in, 5 out]
        n350 = call "Unit Conversion.vi"("환산단위"=w1239, "입력단위"=w1257, "입력값"=w1258) -> ("환산단위"=w1236:string, "환산값 (DBL)"=w1235:dbl, "환산값 (string)"=w1248:string)  [unwired: 3 in, 3 out]
        n351 = call "Unit Conversion.vi"("환산단위"=w1239, "입력단위"=w1255, "입력값"=w1256) -> ("환산값 (string)"=w1247:string)  [unwired: 3 in, 5 out]
        n352 = call "Unit Conversion.vi"("환산단위"=w1239, "입력단위"=w1244, "입력값"=w1254) -> ("환산값 (string)"=w1246:string)  [unwired: 3 in, 5 out]
        n353 = call "Unit Conversion.vi"("환산단위"=w1239, "입력단위"=w1240, "입력값"=w1241) -> ("환산값 (DBL)"=w1234:dbl, "환산값 (string)"=w1237:string)  [unwired: 3 in, 4 out]
        n354 = Replace Array Subset(array=w1253, new element #1=w1250, index #1=13 ("인덱스"), new element #2=w1249, new element #3=w1248, new element #4=w1236, new element #5=w1247, new element #6=w1236, new element #7=w1246, new element #8=w1236, index #8=21 ("인덱스"), new element #9=w1237, index #9=24 ("인덱스"), new element #10=w1236) -> (w1252:string[])  [unwired: 7 in]
      }
      n355 = for {
        shift-right: [w1269] -> w1219
        shift-left: w1226 -> [w1270]
        tunnel: string[] ["Tare", "Tare_Push", "Tare_Pull"] -> [w1267] mode=indexing
        n356 = call-poly "Data Classification.vi"("삭제?(F)"=TRUE, "인덱스"=5, "DATA 입력"=w1270, "검색 문자열"=w1267) -> ("DATA 출력"=w1269:string[][])  [unwired: 3 in, 4 out]
      }
      n357 = Divide(x=w1197, y=2.0) -> (x/y=w1195:dbl)
      n358 = Add(x=w1194, y=w1195) -> (x+y=w1193:dbl)
      n359 = call "Create File Path.vi"("파일타입"=Cmd_File_Type."CSV", "항목"=Cmd_File_path."데이터파일경로", "에러 입력"=w1192, "문자열 in"="Torque Weight Set" ("delimiter (\\t)")) -> ("error out"=w1187:errorcluster, "파일경로"=w1188:path)  [unwired: 4 in, 2 out]
      n360 = call-poly <vilib>:"Read Delimited Spreadsheet.vi"("file path (dialog if empty)"=w1188, "delimiter (\\t)"="," ("delimiter (\\t)")) -> ("all rows"=w1186:string[][])  [unwired: 8 in, 5 out]
      n361 = Index Array(array=w1186, index (col)=w1220) -> (element=w1225:string[])  [unwired: 1 in]
      n362 = call-poly "Data Classification.vi"("인덱스"=2, "DATA 입력"=w1186, "검색 문자열"=w1212) -> ("DATA 출력"=w1222:string[][])  [unwired: 4 in, 4 out]
      n363 = call-poly "Array Deduplication.vi"("배열 in"=w1225) -> ("배열 out"=w1224:string[])  [unwired: 9 in, 1 out]
      n364 = for {
        tunnel: w1224 -> [w1264] mode=indexing
        tunnel: [w1265] -> w1221 mode=indexing
        tunnel: w1222 -> [w1263]
        tunnel: w1220 -> [w1262]
        n365 = call-poly "Data Classification.vi"("인덱스"=w1262, "DATA 입력"=w1263, "검색 문자열"=w1264) -> ("DATA 출력"=w1265:string[][])  [unwired: 4 in, 4 out]
      }
      n366 = call-poly "Data Sorting.vi"("기준열"=u16 3, "Data in"=w1201) -> ("Data out"=w1200:string[][])  [unwired: 8 in, 1 out]
      n367 = call "Variables Data IO.vi"("Select"=Cmd_Var_Data_IO."Resolution", "error in"=w1187, "Func_ext"=w1206) -> ("error out"=w1198:errorcluster, "Data Out"=w1208:string[][], "Func_ext Out"=w1205:string)  [unwired: 6 in]
      n368 = call "Calcu_Torque Weight.vi"("Resolution"=w1208, "Weight Set"=w1221, "torque arm"=w1193, "STD Data"=w1219, "Condition"=w1233) -> ("기타정보"=w1202:string[][], "Condition Out"=w1207:string[][], "분동조합"=w1210:string[][], "분동질량(kg)"=w1211:string[][])  [unwired: 3 in]
      n369 = Insert Into Array(array=w1200, new element=w1202) -> (w1199:string[][])  [unwired: 2 in]
      n370 = call "Variables Data IO.vi"("Write blank data ?(F)"=w1215, "Select"=Cmd_Var_Data_IO."STD3", "error in"=w1198, "Data In"=w1199, "Func_ext"=w1205) -> ("error out"=w1203:errorcluster, "Func_ext Out"=w1204:string)  [unwired: 4 in, 1 out]
      n371 = call "Variables Data IO.vi"("Write blank data ?(F)"=w1215, "Select"=Cmd_Var_Data_IO."STD2", "error in"=w1203, "Data In"=w1210, "Func_ext"=w1204) -> ("error out"=w1217:errorcluster)  [unwired: 4 in, 2 out]
    }
    frame "Torque_2" {
      w1284 = 3 ("인덱스")
      n372 = Index Array(array=w1279, index (col)=2 ("비활성화된 인덱스 (열)")) -> (element=w1311:string[])  [unwired: 1 in]
      n373 = call-poly "Data Classification.vi"("인덱스"=w1284, "DATA 입력"=w1281, "검색 문자열"="반시계방향") -> ("DATA 출력"=w1283:string[][])  [unwired: 4 in, 4 out]
      n374 = call-poly "Data Classification.vi"("인덱스"=w1284, "DATA 입력"=w1281, "검색 문자열"="시계방향") -> ("DATA 출력"=w1286:string[][])  [unwired: 4 in, 4 out]
      n375 = Fract/Exp String To Number(string=w1311) -> (number=w1310:dbl[])  [unwired: 3 in, 1 out]
      n376 = for {
        tunnel: w1310 -> [w1321] mode=indexing
        tunnel: w1286 -> [w1323]
        tunnel: [w1322] -> w1316 mode=indexing
        tunnel: w1283 -> [w1320]
        tunnel: [w1319] -> w1282 mode=indexing
        n377 = for {
          tunnel: w1323 -> [w1332] mode=indexing
          tunnel: [w1327] -> w1322
          tunnel: w1321 -> [w1335]
          tunnel: [w1325] -> w1319
          tunnel: w1320 -> [w1324] mode=indexing
          stop <- w1326 continue-if-true
          n378 = Index Array(array=w1332, index=13 ("인덱스")) -> (element=w1330:string)
          n379 = Fract/Exp String To Number(string=w1330) -> (number=w1329:dbl)  [unwired: 3 in, 1 out]
          n380 = Multiply(x=w1329, y=0.1) -> (x*y=w1328:dbl)
          n381 = Equal To 0?(x=w1335) -> (x = 0?=w1334:bool)
          n382 = In Range and Coerce(upper limit=w1329, x=w1335, lower limit=w1328) -> (In Range?=w1337:bool)  [unwired: 1 out]
          n383 = Or(x=w1334, y=w1337) -> (x .or. y?=w1336:bool)
          n384 = case shown="참" w1336 {
            tunnel: w1332 -> [_ w1339]
            tunnel: [_ w1339] -> w1327
            tunnel: [_ w1338] -> w1325
            tunnel: w1324 -> [_ w1338]
            frame False {
            }
            frame True {
            }
          }
          n385 = Empty Array?(array=w1327) -> (empty?=w1326:bool)
        }
      }
      n386 = Index Array(array=w1281) -> (element=w1277:string[])  [unwired: 2 in]
      n387 = Index Array(array=w1277, index=25 ("인덱스")) -> (element=w1271:string)
      n388 = Index Array(array=w1279, index (col)=2 ("인덱스")) -> (element=w1278:string[])  [unwired: 1 in]
      n389 = Fract/Exp String To Number(string=w1278) -> (number=w1276:dbl[])  [unwired: 3 in, 1 out]
      n390 = call "Number Format.vi"("입력값"=w1271) -> ("정밀도(단위적용)"=w1275:i32)  [unwired: 10 in]
      n391 = Number To Fractional String(number=w1276, precision (6)=w1275) -> (F-format string=w1274:string[])  [unwired: 2 in]
      n392 = Insert Into Array(array=w1274, new element=w1271) -> (w1272:string[])  [unwired: 1 in]
      n393 = call "Variables Data IO.vi"("Write blank data ?(F)"=TRUE ("Write blank data ?(T)"), "Select"=Cmd_Var_Data_IO."STD2", "error in"=w1315, "Data In"=w1282, "Func_ext"=w1313) -> ("error out"=w1289:errorcluster, "Func_ext Out"=w1288:string)  [unwired: 4 in, 1 out]
      n394 = global read "Global_Cal Info.vi" "Func List"() -> (w1296:string[][])
      n395 = global read "Global_Cal Info.vi" "Spec변경?"() -> (w1300:bool[])
      n396 = Index Array(array=w1296, index (col)=2 ("비활성화된 인덱스 (열)")) -> (element=w1298:string[])  [unwired: 1 in]
      n397 = Index Array(array=w1316, index (col)=25 ("인덱스 (행)")) -> (element=w1306:string[])  [unwired: 1 in]
      n398 = Search 1D Array(1D array=w1298, element=w1288) -> (index of element=w1299:i32)  [unwired: 1 in]
      n399 = for {
        tunnel: [w1317] -> w1303 mode=indexing
        tunnel: w1306 -> [w1318] mode=indexing
        n400 = Build Array(w1318, w1318, w1318) -> (w1317:string[])
      }
      n401 = Index Array(array=w1300, index=w1299) -> (element=w1295:bool)
      n402 = Select(t=Cmd_Var_Data_IO."Spec Old" ("Select"), s=w1295, f=Cmd_Var_Data_IO."Spec Default" ("Select")) -> (s? t:f=w1292:T1)
      n403 = call "Variables Data IO.vi"("Select"=w1292, "error in"=w1289, "Func_ext"=w1288) -> ("error out"=w1309:errorcluster, "Data Out"=w1305:string[][], "Func_ext Out"=w1307:string)  [unwired: 6 in]
      n404 = call "Spec Calculation.vi"("기준값 열번호"=2 ("열번호(기준값)"), "Resolution"=w1303, "Condition in"=w1279, "Spec Default"=w1305) -> ("Spec out"=w1301:string[][])  [unwired: 6 in, 1 out]
      n405 = call "Variables Data IO.vi"("Select"=Cmd_Var_Data_IO."Spec", "error in"=w1309, "Data In"=w1301, "Func_ext"=w1307) -> ("error out"=w1314:errorcluster)  [unwired: 5 in, 2 out]
    }
    frame Default {
      w1341 = string[][] [] ("Data out")
    }
  }
  "Cal STD" <- w27
  "Data Out" <- w33
  "Data Out 2" <- w5
  n406 = for {
    tunnel: w26 -> [w1346] mode=indexing
    tunnel: [w1343] -> w17 mode=indexing
    n407 = Concatenate Strings(w1346) -> (w1345:string)
    n408 = call <vilib>:"Trim Whitespace.vi"("string"=w1345) -> ("trimmed string"=w1344:string)  [unwired: 1 in]
    n409 = Empty String/Path?(string/path=w1344) -> (empty?=w1343:bool)
  }
  n410 = Empty Array?(array=w27) -> (empty?=w28:bool)
  "생성오류?" <- w28
  n411 = call "Variables Data IO.vi"("Write blank data ?(F)"=TRUE ("Write blank data ?(T)"), "Select"=Cmd_Var_Data_IO."STD1", "error in"=w36, "Data In"=w27, "Func_ext"=w2) -> ("error out"=→"error out":errorcluster, "Func_ext Out"=→"Func_ext Out":string)  [unwired: 4 in, 1 out]
  n412 = Or Array Elements(Boolean array=w17) -> (logical OR=w16:bool)
  "데이터오류?" <- w16
  n413 = Build Array(w28, w16) -> (w11:bool[])
  n414 = global read "Global_Cal Info.vi" "Func List"() -> (w15:string[][])
  n415 = global read "Global_Cal Info.vi" "std error?"() -> (w12:bool[][])
  n416 = Index Array(array=w15, index (col)=2 ("비활성화된 인덱스 (열)")) -> (element=w14:string[])  [unwired: 1 in]
  n417 = Search 1D Array(1D array=w14, element=w2) -> (index of element=w1:i32)  [unwired: 1 in]
  n418 = Replace Array Subset(array=w12, new element=w11, index (row)=w1) -> (w10:bool[][])  [unwired: 1 in]
  n419 = global write "Global_Cal Info.vi" "std error?"(w10) -> ()
